vi "Doktorarbeit_Cornelius_1.10.vi"(0 "PID 1 COM":refnum<visa-resource-name>="COM3", 1 "Setpoint\n START":bool, 2 "Write to File":bool, 3 "SP 1 input (°C)":dbl=20.0 min=0.0 max=1300.0, 4 "Intervall (s)":u32=1 max=600 format="%.2f", 5 "Write/\nRead":bool=TRUE, 6 "Delay (ms)":u32=500 min=100 max=600000, 7 "Auto Tune":bool, 9 "Standby":bool, 11 "Reset\nSTOPP":bool, 12 "ON":bool caption="OFF", 13 "Get Values":bool, 15 "File Path":path) -> (8 "(°C)":dbl format="%#.3f", 14 "SP 1 is (°C)":dbl)   [LabVIEW 2010]
doc: "1. Verwendung\n\nDas Programm dient der Steuerung und Abfrage des Thermocontrollers I3252 und dem Auslesen von zwei VC 840 Messgeräten und einem Druckmessgerät Pfeiffer Single Gauge. \nDie Messgeräte werden Standardmäßig ausgelesen und erst nach Betätigung des Schalters \"Write to File\" in einer Textdatei abgespeichert. Das Eingabefeld \"Intervall\" legt den Abstand der Messpunkte fest.\nDer Setpoint für den Thermocontroller wird erst nach Betätigung des Tasters \"Setpoint START\" übernommen und angesteuert. Er wird ind den EEPROM des Gerätes geschrieben. Die Regelung kann mit Hilfe des Schalters \"Standby\" unterbrochen werden. Durch den Taster \"Reset STOPP\" kann der Setpoint aus dem EEPROM gelöscht werden.\nDie Eingabeflächen \"Constant\" und \"Thickness\" dienen der Berechnung des spezifischen Widerstands.\nDie Eingabeflächen \"User\" und \"Sample\" werden in den Header der Textdatei übernommen.\nDer Indikator \"File Path\" zeigt den aktuellen Speicherort der Textdatei an. Dieser wird nach ausschalten des Schalters \"Write to File\" gelöscht. Bei erneuten Schreiben muss ein neuer Speicherort gewählt werden. Bei Wahl desselben Speicherorts werden sämtliche bereits gespeicherte Daten gelöscht.\n\n\n2. Erläuterungen zum Blockdiagramm\n2.1 äußere Sequenz\nDie äußerte Sequenz besteht aus fünf Frames. Der erste dient der Initialisierung der Ports. Der zweite dient als Verzögerung um dem Programm genug Zeit zu geben die Ports zu öffnen. Jedoch senden die beiden VC 840 bereits Informationen an den Computer die in einem Puffer zwischengespeichert werden. Im dritten Frame wird dieser Puffer geleert. Somit kommt es zu keinem Framing Error. Desweiteren wird in diesem Frame die Startzeit der Messungen genommen. Im vierten Frame wird die eigentliche Messung und Verarbeitung der Daten durchgeführt. Die while-Schleife wird nur durch Auftreten eines Fehlers oder durch Betätigung des Stopbuttons auf dem Front Panel in der oberen linken Ecke unterbrochen. Im fünften und letzten Frame werden die Ports wieder geschlossen und beim Auftreten eines Fehlers wird das Programm automatisch gestoppt. Falls kein Fehler auftritt wird die Sequenz von vorne abgearbeitet.\n\n2.2 while-Schleife und innere Sequenz\n2.2.1 \"Event Structure\"\n2.2.1.1 Allgemein\nDer erste Frame beinhaltet ein \"Event Structure\". Dieser reagiert auf insgesamt elf verschiedene Ereignisse. Falls keines dieser Ereignisse auftreten sollte, warte die Struktur eine Millisekunde bevor die \"Event Structure\" verlassen wird. Die übrigen Ereignisse treten ein, wenn der entsprechende Kontroller eine Werteänderung erfährt.\n\n2.2.1.2 Event: Setpoint\nDieser Case besteht von außen nach innen aus einer Stacked Sequence, einer for-Loop und einer Flat Sequence die wiederum zwei \"Case Structures\" enthält. Als erstes wird bei dem Schalter \"Setpoint START\" der Blinkmodus aktiviert und bei dem Schalter \"Read Temperature\" deaktiviert. Danach folgt das eigentliche setzen des Temperatursollwerts. In der ersten Iteration wird dem Controller I3252 ein Schreibbefehl gesendet. Theoretisch kann der Setpoint in den RAM oder in den EEPROM geschrieben werden. Diese Auswahl erfolgt mit Hilfe des Schalters \"RAM\". Da das Schreiben in den RAM -Speicher aber aus diversen Gründen nicht erwünscht ist, wurde es nicht implementiert. Eine nachträgliche Implementierung ist aber leicht möglich, in dem die untere String-Konstante \"*P012\" durch \"*W012\" ersetzt wird. An diesem Befehl wird eine fünfstellige Hexadezimalzahl angehängt, die den Sollwert wiedergibt. Der Sollwert wird vorher mit zehn multipliziert, da das Komma standardmäßig nach der ersten Ziffer festgesetzt wurde (Bsp.: 800 wird gesendet um 80 einzustellen). Dieser Befehlsstrang wird an das Gerät mittels des SubVIs \"Comm_Interface\", auf welches später noch näher eingegangen wird, weitergegeben. Der durch das Gerät zurückgegebene String wird nicht verarbeitet.\nDie zweite Iteration dient dem Auslesen des eingestellten Sollwertes. Wahlweise kann der RAM- oder der EEPROM-Speicher ausgelesen werden. Die eigentliche Verarbeitung des Ausgabestrings erfolgt durch das SubVI \"Edit Setpoint\".\nDie Implementierung zur Einstellung des zweiten Setpoints erfolgt durch kopieren der ersten beiden Fälle und ersetzen der \"1\" im Befehf durch eine \"2\" (Bsp.: \"*P012\" zu \"*P022\"). Es darf aber nicht vergessen werden, dass dann ebenfalls die Anzahl der Iterationen angepasst werden muss.\nAls letztes wird der Blinkmodus des Schalters \"Setpoint START\" wieder deaktiviert.\n\n2.2.1.3 Event: Standby\nDieses Ereignis aktiviert bzw. deaktiviert als erstes den Blinckmodus des entsprechenden Schalters und sendet danach den Befehl zum aktivieren (\"*D03\") oder zum deaktivieren (\"*E03\") des Standbymodus an den Thermocontroller.\n\n2.2.1.4 Event: Set Command \nDer in das Feld \"Command shall be\" eingegebene Befehl wird an den Thermocontroller übermittlet. Die korrekte Form des Befehls ist im \"Communication Manuel\" nachzuschlagen. Das \"*\"-Zeichen wurde allerdings schon implementiert und muss somit nicht mit eingegeben werden.\n\n2.2.1.5 Event: Reset\nIn der ersten Iteration wird der Reset-Befehl an den Thermocontroller gesendet. In Folge wird der gesamte EEPROM-Speicher gelöscht. Deshalb wird in der zweiten Iteration der Setpoint aktualisiert. Dieser Befehl hat keinen Einfluss auf den RAM-Speicher. Die anschließende Wartezeit ist auf vier Sekunden festgesetzt und wurde empirisch ermittelt. Diese Zeit benötigt das Gerät um den Reset durchzuführen und für die Kommunikation wieder zur Verfügung zu stehen.\n\n2.2.1.6 Event: Auto Tune\nEs ist festgeschrieben, dass der Setpoint für die \"Auto Tune\"-Funktion wenigstens 20°C über der aktuellen Temperatur liegt. Deshalb wird zunächst der aktuelle Temperaturwert ausgelesen. Im zweiten Schritt werden zu diesem Wert zwanzig addiert und der Setpoint wird in den RAM-Speicher geschrieben. Das Schreiben in diesen Speicher ist nötig, da die \"Auto Tune\"-Funktion\" erst nach einem Reset startet. Im dritten Schritt wird der eigentliche Befehl für den \"Auto Tune\" gesendet (siehe dazu \"Communication Manuel\" S.27). Als vierte und letzte Iteration der for-Schleife folgt der bereits erwähnte Reset-Befehl. Der Temperatursollwert, der im RAM-Speicher eingetragen ist, muss zum Schluss wieder auf 0°C gesetzt werden. Die Zeit für die Ausführung des \"Auto Tune\"-Befehls wurde empirisch ermittelt und 45 s festgesetzt.\n\n2.2.1.7 Event: Write LOW/HI\nDieses Ereignis setzt die am Analogausgang anliegende Spannung fest. Normalerweise beträgt dieser Spannungswert 0-10 V. Das angeschlossene Netzteil verträgt aber maximal nur 2,3 V. Aus diesem Grund wird der \"%HIGH\" auf 23 gesetzt. Somit beträgt die maximal anliegende Spannung nur noch 23% von der maximal möglichen, d.h 2,3V. Ein niedrigerer Wert ist jederzeit möglich, genauso wie ein höherer für den Parameter \"%LOW\". Diese werden zunächst nacheinander in den RAM-Speicher geschrieben und anschließend wieder ausgelesen.\n\n2.2.1.8 Event: Set PID\nDie Werte für den PID-Regler können sowohl mit Hilfe der \"Auto Tune\"-Funktion, als auch manuell eingestellt werden. Es wird wiederum zwischen dem Schreiben in den RAM- und dem EEPROM-Speicher unterschieden. Zunächst werden die Werte für \"P\", \"I\" und \"D\", in dieser Reihenfolge, gesetzt und danach die aktuellen Werte ausgelesen.\n\n2.2.1.9 Event: Get Values\nDieses Ereignis hat zur Folge, dass die Werte für \"P\", \"I\", \"D\", \"%LOW\", \"%HIGH\" und des Setpoints wahlweise aus dem RAM- oder EEPROM-Speicher gelesen werden. Die aktuellen Werte werden nicht nur in die entsprechenden Anzeigefelder übernommen, sondern auch in die entsprechenden Eingabefelder, mit Ausnahme des Temperatursollwerts. \n\n2.2.1.10 Event: RAM\nPrinzipiell kann zwischen dem Schreiben in den RAM- oder EEPROM-Speicher des Thermocontrollers gewählt werden. Die entsprechende Schalterposition auf dem Frontpanel zeigt den aktuell verwendeten Speicher an. Die Anzeigewerte werden bei jedem Umschalten aktualisiert und sind im entsprechenden Speicher eingetragen. Die Implementierung ist identisch mit der des Ereignisses \"Get Values\". Es gilt zu beachten, dass die Werte für \"%LOW\" und \"%HIGH\" nur in den RAM-Speicher geschrieben werden können und somit auch nur aus diesem ausgelesen werden können.\n\n2.2.1.11 Event: Set Gauge to Zero\nMit Hilfe der SubVIs \"Get Pressure\" und \"Offset Display\" werden die Werte für den alten und den neuen Offset und der durch den zweiten Drucksensor ermittelt Druck ermittelt. \n\n2.2.1.12 Event: Write to File\nSollte der Schalter \"Write to File\" aktiviert werden, d.h. Schalterposition oben, so wird zunächst durch das SubVI \"Header\" ein Header für die unter \"File Path\" definierte Datei angelegt. Alle Werte, die bereits in der entsprechenden Datei stehen, werden dabei gelöscht.\n\n2.2.2 \"Timed Structures\"\nIm dritten Frame der inneren Sequenz werden die Werte für Zeitpunkt, Temperatur, Spannung, Strom und Druck ermittelt. Damit die Werte zum gleichen Zeitpunkt aufgenommen werden, werden \"Timed Sequences\" eingesetzt. Mit dem entsprechenden Schalter auf dem Front Panel unter dem Tab \"Settings\" kann gewählt werden, ob das entsprechende Gerät ausgelesen werden soll oder nicht. Die einzelnen Sequenzen werden parallel abgearbeitet, womit die Prozesszeit von diesem Frame durch der zeitintensivsten Sequenz abhängt. Dies ist in aller Regel das Auslesen der Temperatur, da ein \"Delay\" von 500 ms oder größer benötigt wird, um den Controller ordentlich ansprechen zu können.\nDie Systemzeit wird durch das SubVI \"System Time in Seconds\" in Sekunden umgerechnet und der in dem Parameter \"Starttime\" gespeicherte Wert wird abgezogen. Somit werden die Sekunden seit dem Start des Programms gezählt.\n\n2.2.3 restlichen Frames\nIm zweiten Frame wird das Intervall zwischen den einzelnen Messwerten festgelegt. Dabei wird der Wert des Parameters \"Delay\" abgezogen. Dieser Wert beträgt im Normalfall 500 ms und ist somit nicht vernachlääsigbar.\nDer Vierte Frame beinhaltet die Umrechnung des Temperatur-Strings in einen Temperaturwert durch das SubVI \"Edit Tmperature\", die Berechnung des spezifischen Widerstands durch das SubVI \"Resistivity Calculation\" und die Überprüfung des Druckwerts. Auch werden die neu gewonnen Werte in das entsprechende Shift-Register übernommen. Falls der Druckwert einen in dem Parameter \"Pressure Limit (mbar)\" festgelegten Grenzwert überschreiten sollte, wird der Thermocontroller automatisch in den Standby-Modus versetzt. Des Weiteren wird der Schalter \"Standby\" solange gesperrt, wie der Druck oberhalb des Grenzwertes liegt. Wenn der Druck wieder unter den Grenzwert gesunken ist, wird der Standby-Befehl nicht automatisch aufgehoben, sondern muss vom Benutzer durch Betätigung des entsprechenden Schalters gegeben werden.\nIm fünften Frame werden die Diagramme erstellt. Dabei wird jedes Mal von neuem das gesamte Shift-Register als Graph dargestellt. Weiterhin werden die Messwerte in ein 1D-Array geschrieben.\nDer sechste und letzte Frame beinhaltet den eigentlich Schreibvorgang der Messwerte in eine Textdatei und die Überprüfung ob ein Fehler vorliegt.\n\n2.3 SubVIs\n2.3.1 Allgemein\nDie SubVIs für die Messgeräte VC840 und das Druckmessgerät wurden aus anderen Quellen übernommen. \n\n2.3.2 \"Header\"\nIn den Header wird zunächst das aktuelle Datum und die aktuelle Zeit übernommen. Die ausgewählte Datei wird dabei überschrieben. Danach wird der Name des Benutzers und der Probe übernommen. Zum Schluss werden die Einheiten in einer Reihe, durch einen Tabulator getrennt, in den Header geschrieben.\n\n2.3.3 \"I3252 Comm Interface\"\nDieses VI stellt die Kommunikation mit dem Thermocontroller her und gibt den Ausgabe-String zurück.\n\n2.3.4 \"I3252 Edit Setpoint\"\nIm Ausgabe-String vom Thermocontroller ist an der vierten Stelle die Stelle des Dezimalpunktes verschlüsselt. Dieses Hexadezimalzahl wird herausgefiltert und an ein \"ENUM Controller\" übergeben. Dieser weist der Hexadezimalzahl eine Nummer zu, mit welcher ein Wert aus einem Array entnommen wird. Dieser Wert dient als Quotient. Der tatsächliche Wert kann somit errechnet werden.\n\n2.3.5 \"I3252 Edit Temperature\"\nDer Temperatur-String, der vom Thermocontroller zurückgegeben wird, wird in eine Dezimalzahl umgewandelt. Manchmal kommt es aus zu Dropouts, die durch dieses Programm herausgefiltert werden. Der letzte Wert wird dabei in einer \"Feedback Node\" gehalten unter der Annahme, dass sich der Temperaturwert nicht sprunghaft ändert.\n\n2.3.6 \"Resistivity Calculation\"\nDer spezifische Widerstand wird nach folgender Formel ausgerechnet. Dabei entspricht t der Dicke der Probe und C ist eine Konstante.\nrho=C*pi*t*U/(ln( 2)*I)\n\n2.3.7 \"System Time in Seconds\"\nZunächst wird die aktuelle Systemzeit ausgelesen. Danach wird diese in Stunden, Minuten und Sekunden aufgeteilt, alles in Sekunden umgerechnet und letztendlich addiert."
uses:
  <vilib>/Platform/TimedLoop/XDataNode/XDataNode.xnode
  <vilib>/Platform/TimedLoop/XDataNode/timing_clust.ctl
  <vilib>/Platform/TimedLoop/XDataNode/nitl_modes.ctl
  <vilib>/Platform/TimedLoop/XDataNode/wakeup.ctl
  <vilib>/Instr/_visa.llb/VISA Configure Serial Port (Instr).vi
  <vilib>/Platform/TimedLoop/scheduler/LVUserAPI/_suppVIs/Create_1kHz_TSource.vi
  <vilib>/Utility/file.llb/Write To Spreadsheet File (DBL).vi
  <vilib>/Platform/TimedLoop/XDataNode/XDNodeRunTimeDep.lvlib
  Labview 8 Tutorial/Dual Gauge/Dual Gauge.lvlib
panel:
  out "appended array":dbl[](array[numeric])
  in  "Tab Control":T1(tab)
  in  "Thickness (nm)":dbl min=0.0
  in  "4PP constant":dbl min=0.0 max=5.0
  in  "Sample":string
  in  "User":string
  out "Sample holder (Type-K Thermocouple)":cluster{dbl[], dbl[]}(graph)
  out "current time (s)":dbl
  out "data logger intervall (s)":dbl
  out "loop time (s)":ext
  in  "stop":bool
  out "Main Chamber (PG-1)":cluster{dbl[], dbl[]}(graph)
  out "Pressure Gauge 1#1":dbl format="%#_4e"
  out "Loadlock (PG-3)":cluster{dbl[], dbl[]}(graph)
  out "Pressure Gauge 1#2":dbl format="%#_3e"
  out "Pressure Gauge 2#1":dbl format="%#_3e"
  out "Pressure OpenPort":cluster{dbl[], dbl[]}(graph)
  out "Pressure Gauge 2#2":dbl caption="current"
  out "Pirani (VVP1 Scroll)":cluster{dbl[], dbl[]}(graph)
  out "status 2":bool caption="Status"
  out "code 2":i32 caption="Code"
  out "code":i32 caption="Code"
  out "status":bool caption="Status"
  in  "Set Gauge to Zero":bool
  out "Status Gauge 1#2":i32(ring) items=["data OK", "underrange", "overrange", "sensor error", "sensor off", "no sensor", "ID error"]
  out "Pressure Gauge 1#2":dbl format="%.3e"
  out "Pressure Gauge 1#1":dbl format="%.3e"
  out "Status Gauge 1#1":i32(ring) items=["data OK", "underrange", "overrange", "sensor error", "sensor off", "no sensor", "ID error"]
  in  "TPG 1 COM":refnum<visa-resource-name>="COM1"
  in  "Pressure Limit (mbar)":dbl=1.0 min=0.0 max=1100.0
  out "Current Offset (mbar)":dbl
  in  "ON (TPG 2)":bool caption="OFF"
  in  "ON (TPG 1)":bool=TRUE caption="OFF"
  in  "ON":bool caption="OFF"
  in  "VC 840 2":refnum<visa-resource-name>="COM4"
  out "Reading 2":dbl format="%_4f"
  out "Mode 2":enum16{"?", "Diode", "Beep", "DC", "AC"}(ring)
  out "Unit 2":string
  in  "VC 840 1":refnum<visa-resource-name>="COM4"
  out "Reading 1":dbl format="%_4f"
  out "Mode 1":enum16{"?", "Diode", "Beep", "DC", "AC"}(ring)
  out "Unit 1":string
  out "Status 1":T2
  out "Status 2":T2
  in  "ON":bool caption="OFF"
  out "% HIGH Istwert":u32
  out "% LOW Istwert":u32
  in  "% High Sollwert":u32=23 max=24
  in  "% LOW Sollwert":u32 max=25
  in  "RAM":bool=TRUE caption="EEPROM"
  out "D (Rate) IstWert":u32
  out "I ( Reset1) Istwert":u32
  out "P (PB1) Istwert":u32 caption="actual value"
  in  "D (Rate) Sollwert":u32 max=3999
  in  "I ( Reset1) Sollwert":u32 max=3999
  in  "P (PB1) Sollwert":u32 caption="set value" max=9999
  in  "Set Command":bool
  in  "Set PID":bool
  in  "Write LOW/HI":bool
  in  "Flow Control":u16(ring) items=["None"=0, "XON/XOFF"=1, "RTS/CTS"=2, "DTR/DSR"=4]
  in  "Stop Bits":u16(ring)=10 items=["1.0"=10, "1.5"=15, "2.0"=20]
  in  "Parity":u16(ring)=1 items=["None", "Odd", "Even", "Mark", "Space"]
  in  "Data Bits":u16=7 min=5 max=8 step=1
  in  "Baud Rate":u32=9600
  out "Command output":string
  in  "Command input":string
  in  "TPG 2 COM":refnum<visa-resource-name>="COM4"
  out "Pressure Gauge 2#2":dbl format="%.3e"
  out "Pressure Gauge 2#1":dbl format="%.3e"
  out "Status Gauge 2#2":i32(ring) items=["data OK", "underrange", "overrange", "sensor error", "sensor off", "no sensor", "ID error"]
  out "Status Gauge 2#1":i32(ring) items=["data OK", "underrange", "overrange", "sensor error", "sensor off", "no sensor", "ID error"]
  out "Current":cluster{dbl[], dbl[]}(graph)
  out "Voltage":cluster{dbl[], dbl[]}(graph)
  out "Voltage (V)":dbl format="%.4e"
  out "Current (A)":dbl format="%.4e"
  out "Resistivity":cluster{dbl[], dbl[]}(graph)
  out "Resistivity (Ohm*cm)":dbl format="%.3e"
  # "set \nvalue"
  # "actual \nvalue"
  # "T (°C)"
  # "mbar"
  # "mbar"
  # "mbar"
  # "mbar"
  # "Pressure Measurement \n(Pfeiffer TPG261)"
  # "PID Controller (Omega Newport i3252)"
  # "limit (mbar)"
  # "Multimeter\n#1 (VC 840)"
  # "Multimeter\n#2 (VC 840)"
  # "P"
  # "I"
  # "D"
  # "% Low"
  # "% High"
  # "Authors:  Daniel Schuster (sir-dan@web.de)\n                 Steffen Cornelius (s.cornelius@hzdr.de)\n                 Nico Spahn (x)\n\n                 premade SubVIs for readout of Pfeiffer gauge and VC840 Multimeters were used\n                 SubVI \"I3252_Comm_Interface\" is based on a modified Labview example\n\nRelease:  v1.0    \n\nVersion History:\n\nv1.1  -    28.06.2011\n             - Format des Files geändert von %.3f auf %g\n             - maximale Eingabewerte für PID begrenzt\nv1.2  -    12.07.2011\n             - Anzeige p,rho, U, V auf Scientific geändert\n             - y-Achse p,rho auf Log geändert\n             - numerische Zeitanzeige hinzugefügt\n             - 4PP Constant: pi/ln(2)=4,532 set as the default value\nv1.3  -    25.07.2011\n             - Zeitvariable auf EXT geändert, um Sprünge in Diagrammen loszuwerden\nv1.4  -   27.07.2011\n             - ALLE Variablen auf DBL zurückgesetzt wegen Formatierungsproblem im File\n             - Zeitberechnung neu gemacht (Tick count differenzen) -> Zeitsprünge korrigiert ?\n             - Delay/Intervall überarbeitet\nv1.5  -   05.12.2012\n                - Austausch der alten Pfeifer SubvIs durch neue -> nun alle 4 Kanäle des DualGauge\n                                                                                                         Controllers gleichzeitig auslesbar\n                - neue Pfeiffer SubVIs verwendet in Druckwertauslesung und Offset Berechnung des Baratron\n                  Druckes (COM5 Sensor1)\n                - Neuarragement des GUI -> FullRange und Baratron neben Temperatur auf Haupseite zu sehen\n                                                                   Pirani und OpenPort auf Meas.2 zu sehen\n                                                                   Diagnose Seite umfasst nun auch Widerstandsdiagramm\n                - Änderungen der Settingseite -> nun alle 4 Drucksensoren mit aktuellem Messwert und Gerätestatus\n                                                                           zu sehen\n                - The readout of the PID-Temperature Controller and the VC840 Multimeters was not modified\nv1.73  -  18.10.2013\n                - Layout Änderungen\nv.1.8   -  19.01.2014\n                - Änderung Layout Settings Tab\n                - Trennung der beiden TPG Dual Gauge Controls\n                -"
  # "Version 1.73    - last change 18.10.2013"
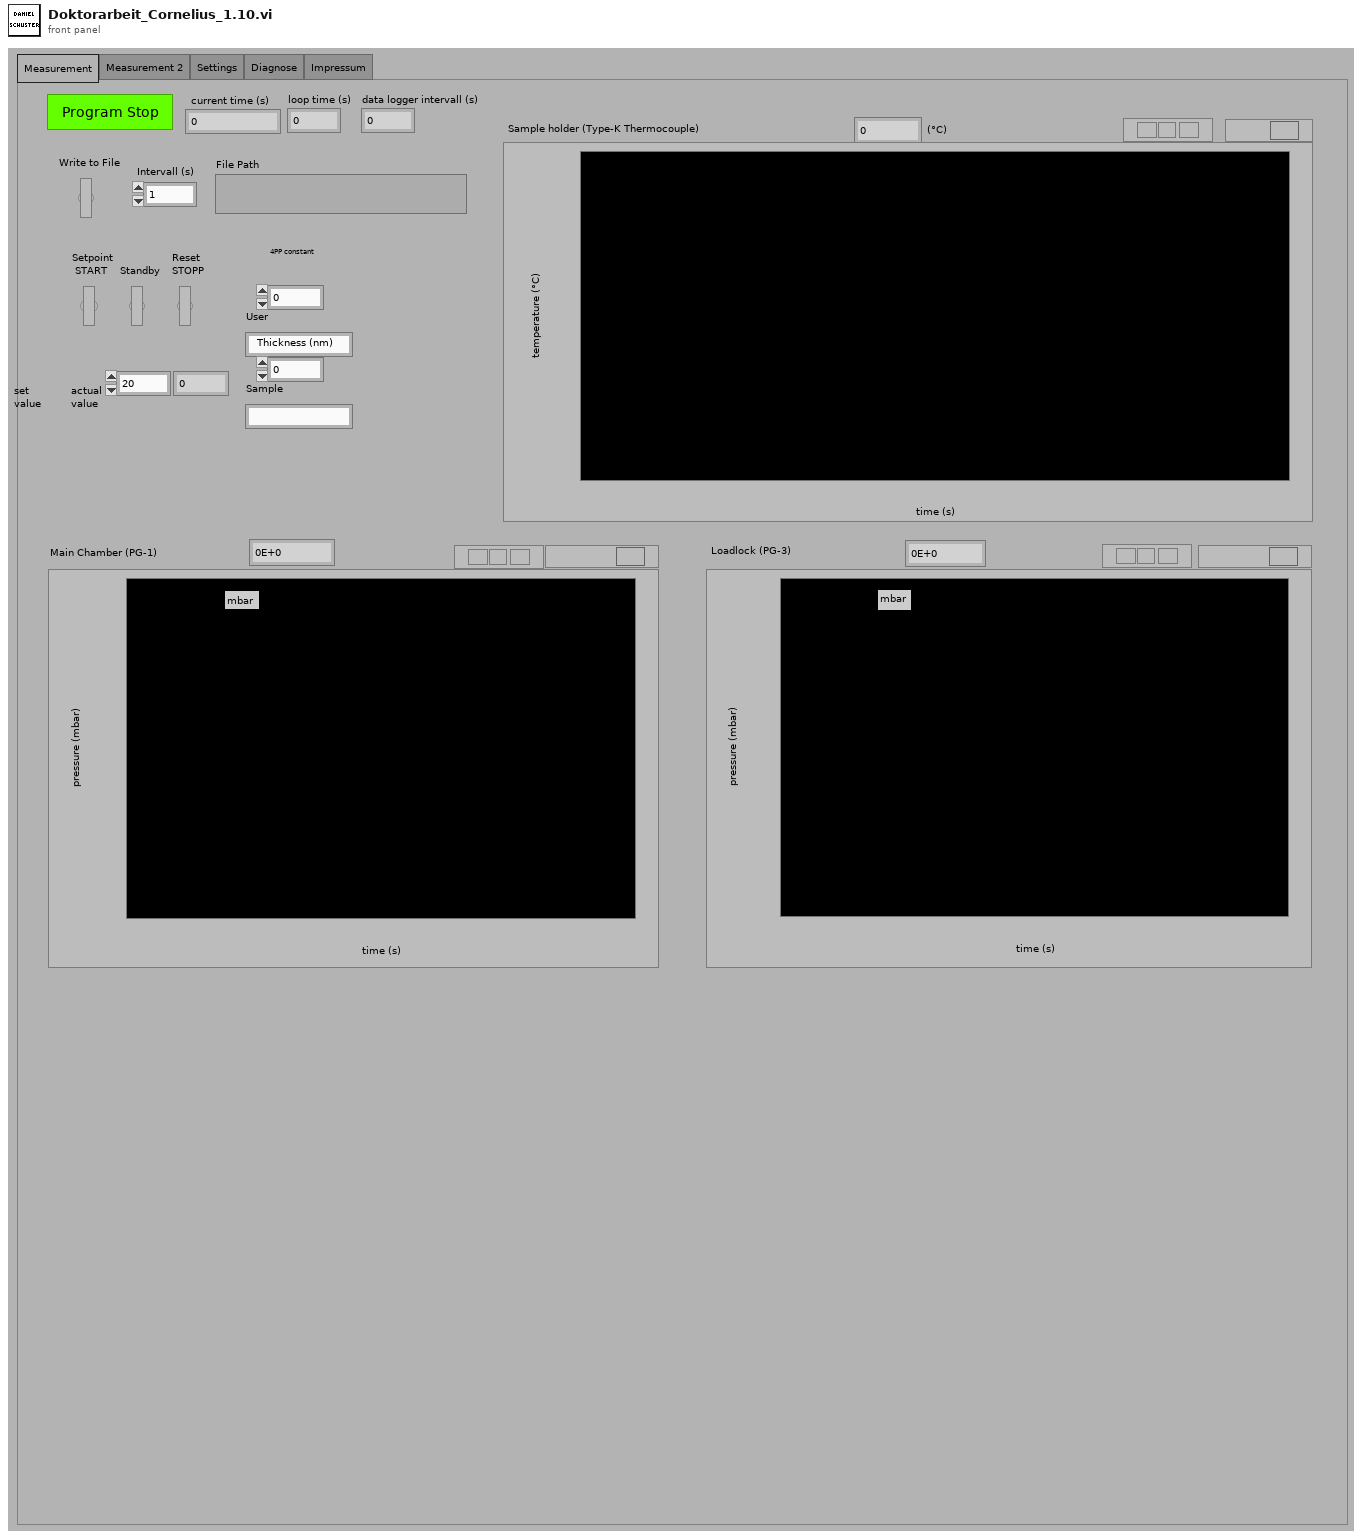
[diagram p1: front panel]
types:
  T1 = enum32{"Measurement", "Measurement 2", "Settings", "Diagnose", "Impressum"}
  T2 = cluster{"Low Bat":bool, "Auto":bool, "Delta":bool, "Hold":bool, "RS232":bool}
  T3 = typedef "XDNodeRunTimeDep.lvlib/timing_clust.ctl" = cluster{"Expected End [f-1]":u64, "Actual End [f-1]":u64, "Finished Late? [f-1]":bool, "Expected End [i-1]":u64, "Actual End [i-1]":u64, "Finished Late? [i-1]":bool, "Expected Start [i]":u64, "Actual Start [i]":u64, "Expected Start [f]":u64, "Actual Start [f]":u64, "Source Name":string, "Structure Name":string, "Period":i64, "Deadline":i64, "Offset":i64, "Start":i64, "Priority":i32, "Timeout":i32, "Mode":T4, "Wakeup Reason":T5, "Error":errorcluster, "Source Type":string, "Secondary Source Type":string, "Global End Time":u64, "Global Start Time":u64, "Frame Duration":u64, "Iteration Duration":u64, "Assigned CPU":i32, "I/O Scan Engine Mode":u32}
  T4 = typedef "XDNodeRunTimeDep.lvlib/nitl_modes.ctl" = enum32{"No Change", "Process missed periods, maintain original phase", "Discard missed periods, maintain original phase", "Process missed periods, ignore original phase", "Discard missed periods, ignore original phase"}
  T5 = typedef "XDNodeRunTimeDep.lvlib/wakeup.ctl" = enum32{"Normal", "Aborted", "Asynchronous wakeup", "Timing source error", "Timed loop error", "Timeout"}
  T6 = enum8{"Enabled", "Disabled", "Disabled and Grayed Out"}
  T7 = cluster{"VISA resource name out":refnum<visa-resource-name>, "error out":errorcluster, "Delay (ms)":u32, "Write/\nRead":bool}
  T8 = cluster{"TPG 2 COM":refnum<visa-resource-name>, "error out":errorcluster}
  T9 = cluster{"COM out":refnum<visa-resource-name>, "Cluster (Ausgang)":errorcluster}
  T10 = cluster{"Pressure Gauge#1":dbl, "Pressure Gauge#2":dbl}
  T11 = cluster{"TPG 1 COM":refnum<visa-resource-name>, "error out":errorcluster}
  T12 = cluster{"COM out":refnum<visa-resource-name>, "error out":errorcluster, "COM out":refnum<visa-resource-name>, "error out":errorcluster}
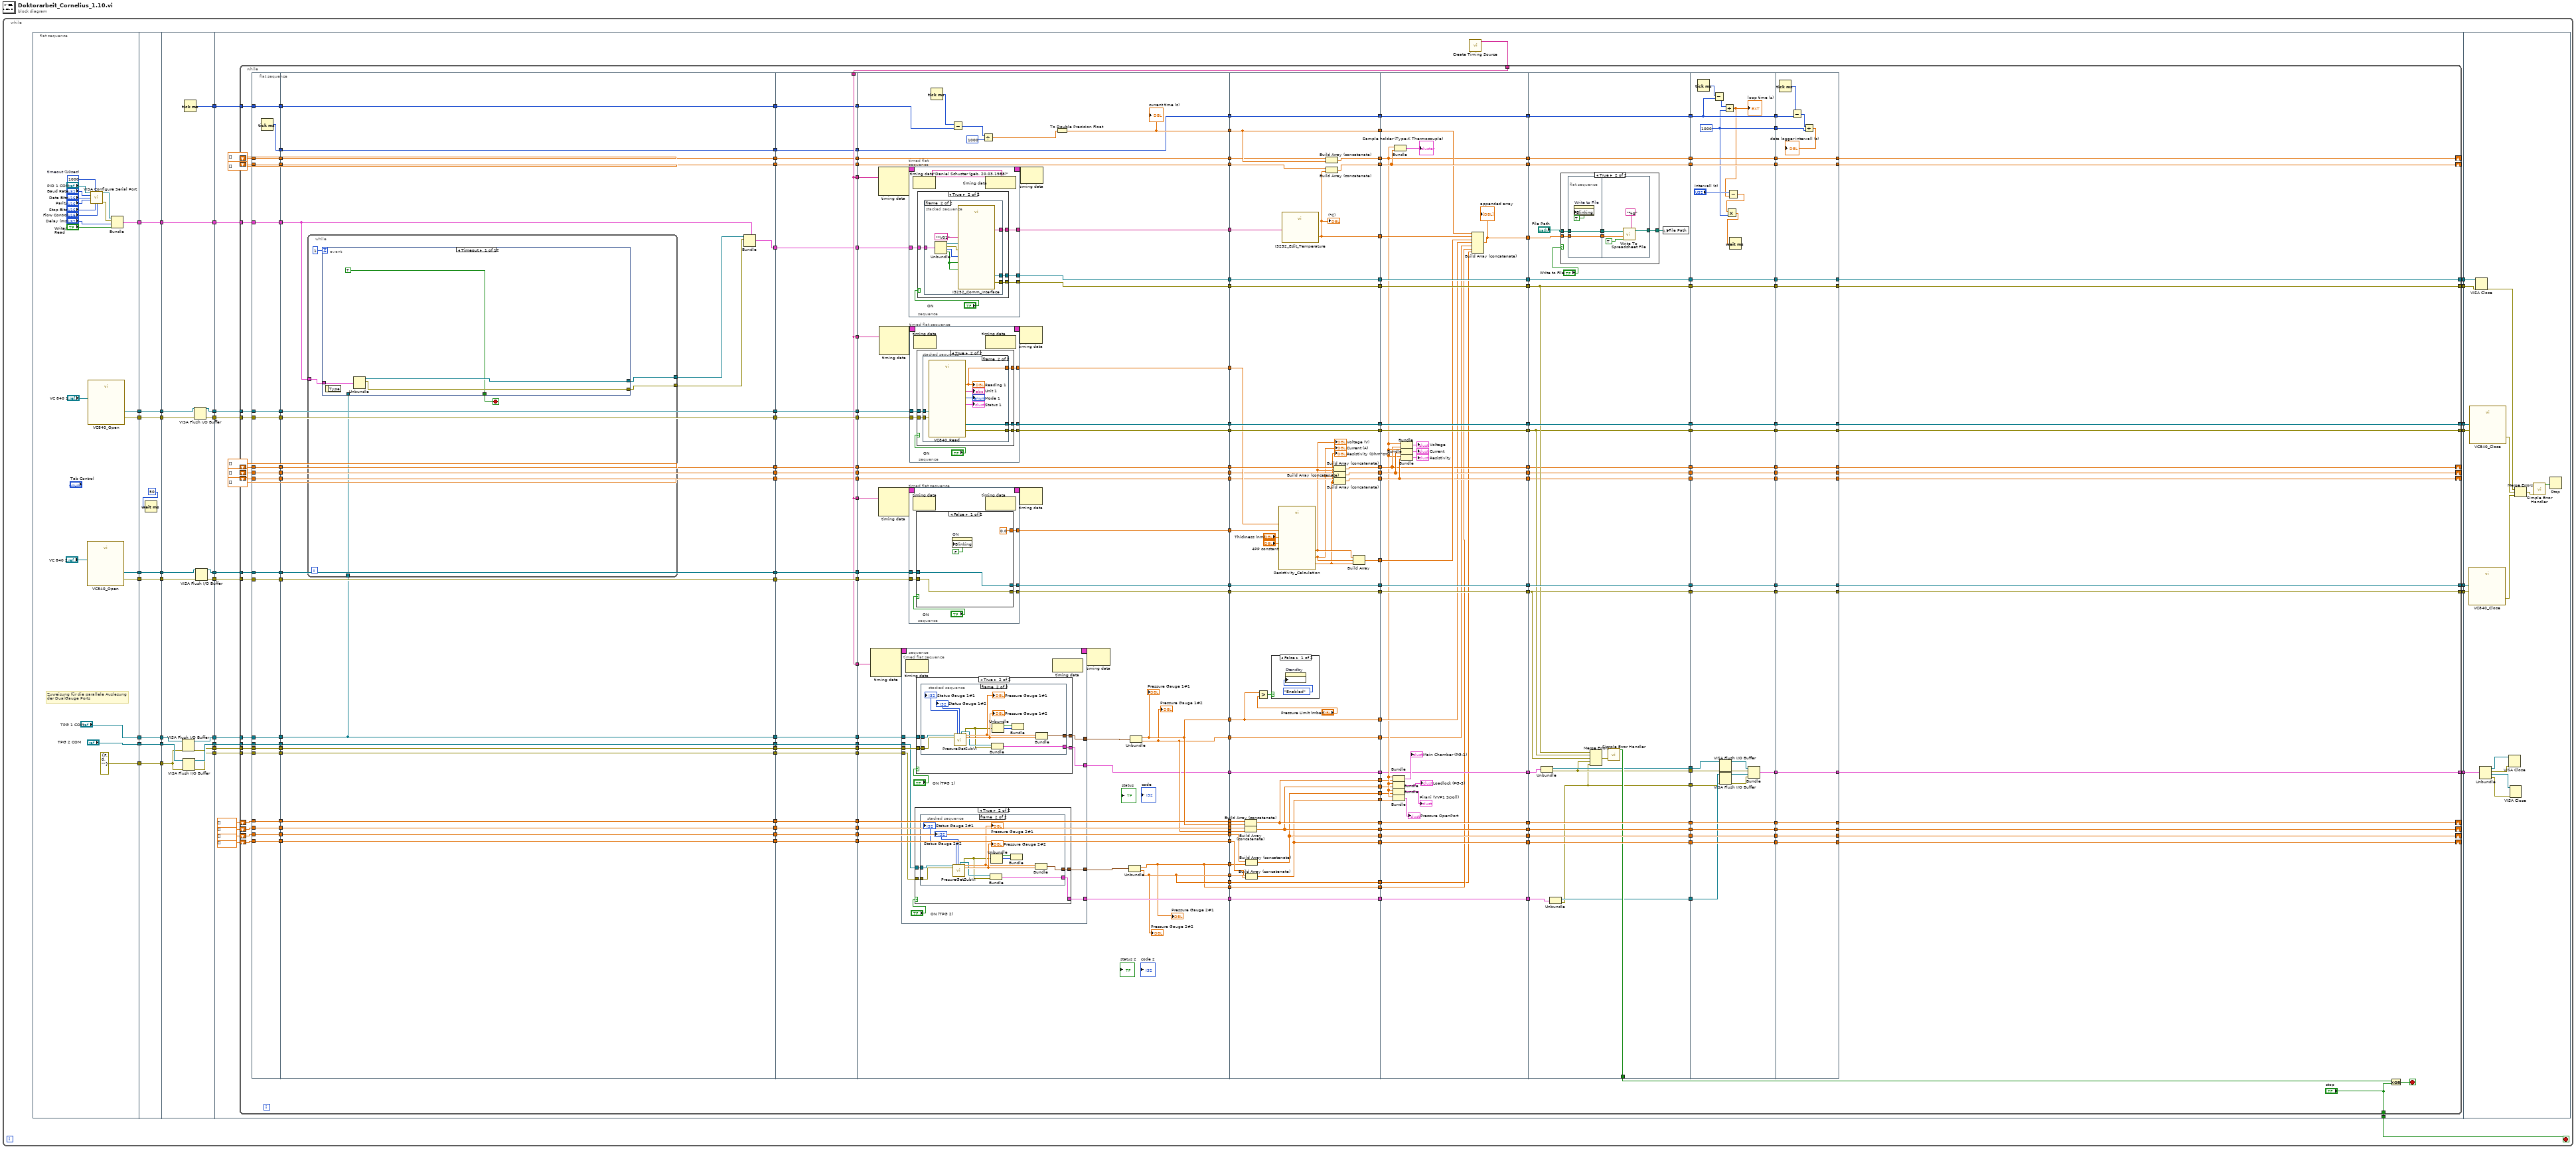
[diagram p0: block diagram]
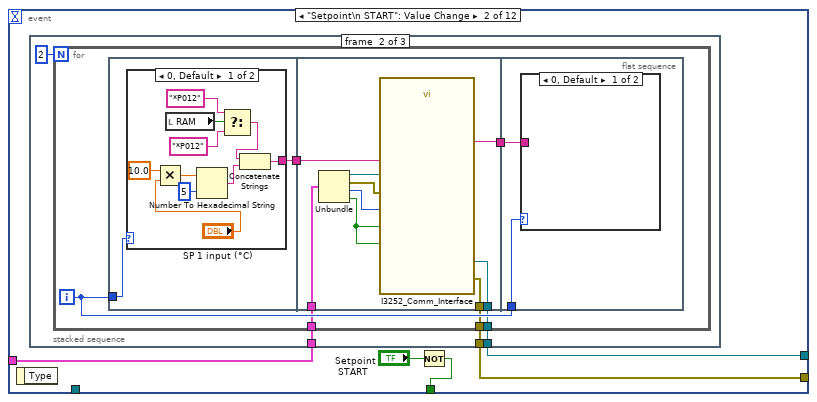
[diagram p2: hidden frame]
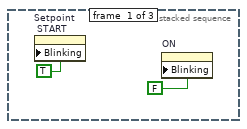
[diagram p3: hidden frame]
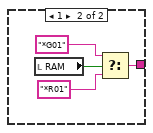
[diagram p4: hidden frame]
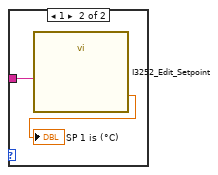
[diagram p5: hidden frame]
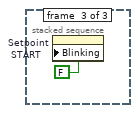
[diagram p6: hidden frame]
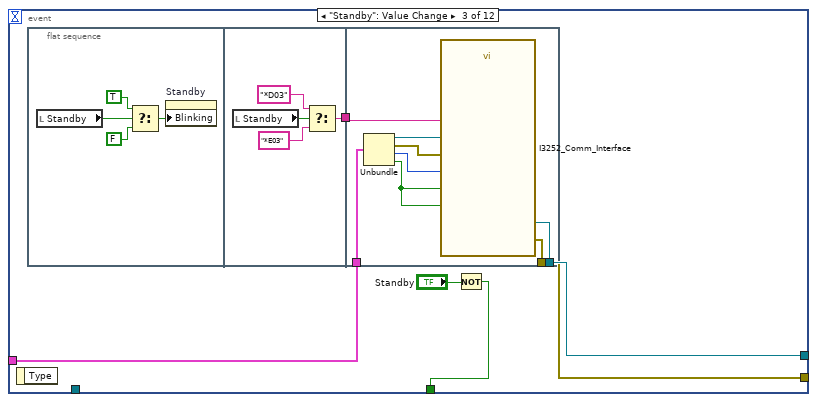
[diagram p7: hidden frame]
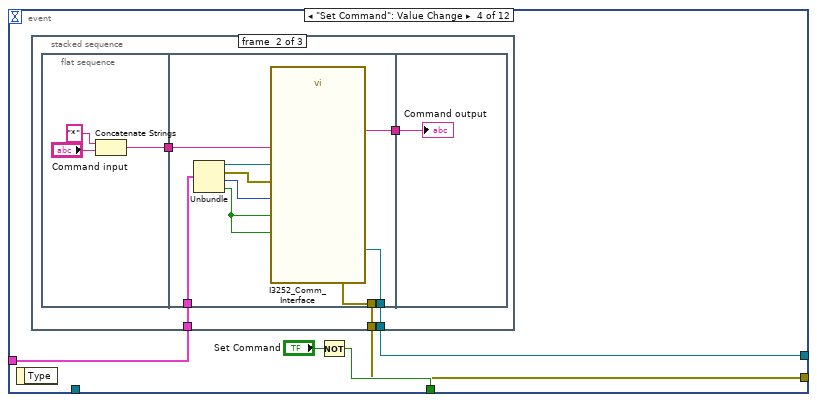
[diagram p8: hidden frame]
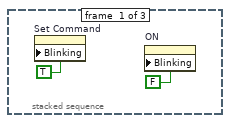
[diagram p9: hidden frame]
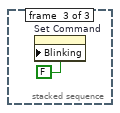
[diagram p10: hidden frame]
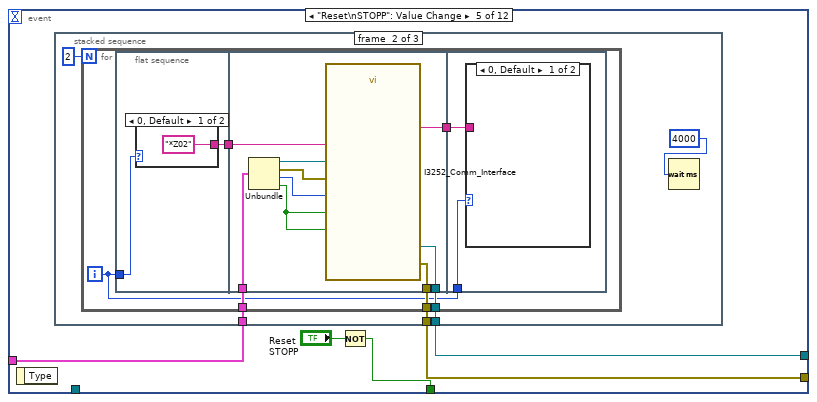
[diagram p11: hidden frame]
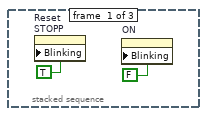
[diagram p12: hidden frame]
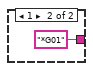
[diagram p13: hidden frame]
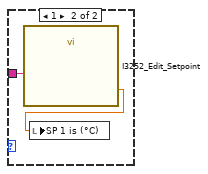
[diagram p14: hidden frame]
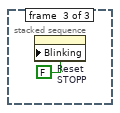
[diagram p15: hidden frame]
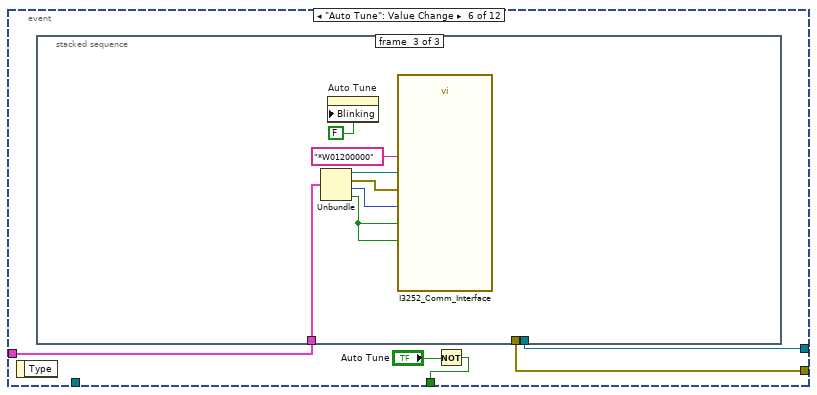
[diagram p16: hidden frame]
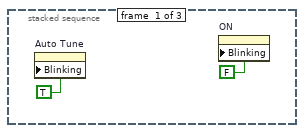
[diagram p17: hidden frame]
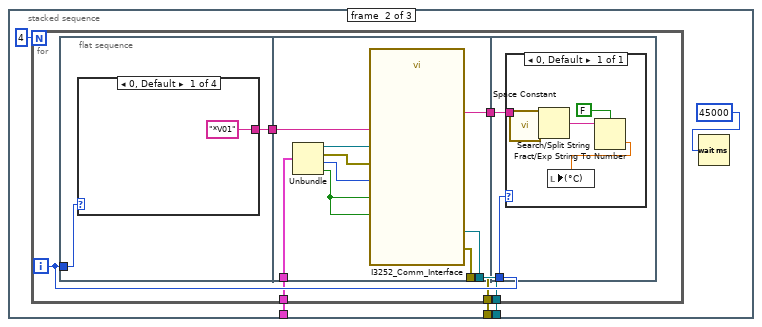
[diagram p18: hidden frame]
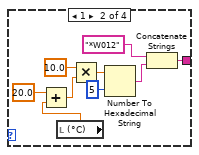
[diagram p19: hidden frame]
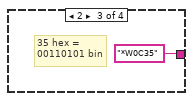
[diagram p20: hidden frame]
diagram:
  n1 = while {
    stop <- w6 stop-if-true
    n2 = flat-sequence {
      tunnel: [w54] -> w34
      tunnel: [w55] -> w33
      tunnel: [w40] -> w32
      tunnel: [w53] -> w31
      tunnel: [w52] -> w30
      tunnel: ["TPG 1 COM"] -> w29
      tunnel: ["TPG 2 COM"] -> w28
      tunnel: [errorcluster {"status"=FALSE, "code"=0, "source"=""} ("Fehler (Eingang)")] -> w3
      tunnel: w34 -> [w64]
      tunnel: [w64] -> w27
      tunnel: w33 -> [w63]
      tunnel: [w63] -> w26
      tunnel: w32 -> [w62]
      tunnel: [w62] -> w25
      tunnel: w31 -> [w61]
      tunnel: [w61] -> w24
      tunnel: w30 -> [w60]
      tunnel: [w60] -> w23
      tunnel: [w58] -> w22
      tunnel: w29 -> [w58]
      tunnel: [w57] -> w21
      tunnel: w28 -> [w57]
      tunnel: [w56] -> w4
      tunnel: w3 -> [w56]
      tunnel: w27 -> [w75]
      tunnel: [w74] -> w20
      tunnel: w26 -> [w76]
      tunnel: [w73] -> w19
      tunnel: w25 -> [w81]
      tunnel: [w81] -> w18
      tunnel: w24 -> [w78]
      tunnel: [w79] -> w17
      tunnel: w23 -> [w77]
      tunnel: [w80] -> w16
      tunnel: [w72] -> w15
      tunnel: [w70] -> w14
      tunnel: w22 -> [w71]
      tunnel: [w69] -> w13
      tunnel: w21 -> [w68]
      tunnel: w4 -> [w67]
      tunnel: [w66] -> w2
      tunnel: [w65] -> w1
      tunnel: w20 -> [w109]
      tunnel: w19 -> [w108]
      tunnel: w18 -> [w107]
      tunnel: w17 -> [w105]
      tunnel: w16 -> [w104]
      tunnel: [w103] -> w12
      tunnel: [w102] -> w11
      tunnel: [w101] -> w10
      tunnel: [w100] -> w9
      tunnel: [w99] -> w8
      tunnel: [w98] -> w7
      tunnel: w15 -> [w92]
      tunnel: w14 -> [w91]
      tunnel: w13 -> [w90]
      tunnel: [w85] -> w6
      tunnel: [w84] -> w5
      tunnel: w2 -> [w83]
      tunnel: w1 -> [w82]
      tunnel: w12 -> [w1315]
      tunnel: w11 -> [w1314]
      tunnel: w10 -> [w1317]
      tunnel: w9 -> [w1316]
      tunnel: w8 -> [w1319]
      tunnel: w7 -> [w1318]
      tunnel: w5 -> [w1312]
      frame #0 {
        w41 = u32 1000  # timeout (10sec)
        # "Zuweisung für die parallele Auslesung\nder DualGauge Ports"
        n3 = call "VC840_Open.vi"("VISA resource name"="VC 840 2") -> ("error out"=w52:errorcluster, "VISA resource name out"=w53:refnum<visa-resource-name>)  [unwired: 1 in, 8 out]
        n4 = call "VC840_Open.vi"("VISA resource name"="VC 840 1") -> ("error out"=w55:errorcluster, "VISA resource name out"=w54:refnum<visa-resource-name>)  [unwired: 1 in, 8 out]
        n5 = call-poly "VISA Configure Serial Port"("VISA resource name"="PID 1 COM", "timeout (10sec)"=w41, "baud rate (9600)"="Baud Rate", "data bits (8)"="Data Bits", "parity (0:none)"="Parity", "stop bits (10: 1 bit)"="Stop Bits", "flow control (0:none)"="Flow Control") -> ("VISA resource name out"=w50:refnum<visa-resource-name>, "error out"=w51:errorcluster)  [unwired: 2 in, 5 out]
        n6 = Bundle("VISA resource name out"=w50, "error out"=w51, "Delay (ms)"="Delay (ms)", "Write/\nRead"="Write/\nRead") -> (w40:T7)  [unwired: 1 in]
      }
      frame #1 {
        n7 = Wait (ms)(milliseconds to wait=u32 50) -> ()  [unwired: 1 out]
      }
      frame #2 {
        n8 = VISA Flush I/O Buffer(VISA resource name=w71, error in (no error)=w67) -> (VISA resource name out=w70:refnum<visa-resource-name>, error out=w66:errorcluster)  [unwired: 1 in]
        n9 = VISA Flush I/O Buffer(VISA resource name=w68, error in (no error)=w67) -> (VISA resource name out=w69:refnum<visa-resource-name>, error out=w65:errorcluster)  [unwired: 1 in]
        n10 = Tick Count (ms)() -> (millisecond timer value=w72:u32)
        n11 = VISA Flush I/O Buffer(VISA resource name=w75, error in (no error)=w76) -> (VISA resource name out=w74:refnum<visa-resource-name>, error out=w73:errorcluster)  [unwired: 1 in]
        n12 = VISA Flush I/O Buffer(VISA resource name=w78, error in (no error)=w77) -> (VISA resource name out=w79:refnum<visa-resource-name>, error out=w80:errorcluster)  [unwired: 1 in]
      }
      frame #3 {
        n13 = call-poly <vilib>:"Create Timing Source.vi"() -> ("name (out)"=w106:string)  [unwired: 10 in, 1 out]
        n14 = while {
          tunnel: w109 -> [w328]
          tunnel: w108 -> [w327]
          tunnel: w107 -> [w326]
          tunnel: w106 -> [w319]
          tunnel: w105 -> [w312]
          tunnel: w104 -> [w311]
          tunnel: [w307] -> w103
          tunnel: [w306] -> w102
          tunnel: [w304] -> w101
          tunnel: [w302] -> w100
          tunnel: [w300] -> w99
          tunnel: [w298] -> w98
          shift-right: [w271] -> _
          shift-left: dbl[] [] -> [w276]
          shift-right: [w249] -> _
          shift-left: dbl[] [] -> [w284]
          shift-right: [w273] -> _
          shift-left: dbl[] [] -> [w280]
          shift-right: [w246] -> _
          shift-left: dbl[] [] -> [w283]
          shift-right: [w243] -> _
          shift-left: dbl[] [] -> [w282]
          tunnel: w92 -> [w237]
          tunnel: w91 -> [w193]
          tunnel: w90 -> [w189]
          shift-right: [w147] -> _
          shift-left: dbl[] [] -> [w177]
          shift-right: [w145] -> _
          shift-left: dbl[] [] -> [w175]
          shift-right: [w143] -> _
          shift-left: dbl[] [] -> [w173]
          shift-right: [w141] -> _
          shift-left: dbl[] [] -> [w171]
          tunnel: ["stop"] -> w85
          tunnel: [w135] -> w84
          tunnel: w83 -> [w130]
          tunnel: w82 -> [w128]
          stop <- w134 stop-if-true
          n15 = flat-sequence {
            tunnel: w237 -> [w338]
            tunnel: w276 -> [w339]
            tunnel: w280 -> [w340]
            tunnel: w282 -> [w341]
            tunnel: w283 -> [w342]
            tunnel: w284 -> [w343]
            tunnel: w311 -> [w344]
            tunnel: w312 -> [w345]
            tunnel: w326 -> [w346]
            tunnel: w327 -> [w347]
            tunnel: w328 -> [w348]
            tunnel: [w348] -> w236
            tunnel: [w347] -> w235
            tunnel: [w346] -> w234
            tunnel: [w345] -> w233
            tunnel: [w344] -> w232
            tunnel: [w343] -> w231
            tunnel: [w342] -> w230
            tunnel: [w341] -> w229
            tunnel: [w340] -> w228
            tunnel: [w339] -> w227
            tunnel: [w338] -> w226
            tunnel: [w337] -> w208
            tunnel: [w336] -> w194
            tunnel: w193 -> [w336]
            tunnel: [w335] -> w190
            tunnel: w189 -> [w335]
            tunnel: [w334] -> w178
            tunnel: w177 -> [w334]
            tunnel: [w333] -> w176
            tunnel: w175 -> [w333]
            tunnel: [w332] -> w174
            tunnel: w173 -> [w332]
            tunnel: [w331] -> w172
            tunnel: w171 -> [w331]
            tunnel: [w330] -> w131
            tunnel: w130 -> [w330]
            tunnel: [w329] -> w129
            tunnel: w128 -> [w329]
            tunnel: [w371] -> w325
            tunnel: [w370] -> w323
            tunnel: [w366] -> w321
            tunnel: [w365] -> w316
            tunnel: [w364] -> w314
            tunnel: [w363] -> w281
            tunnel: [w362] -> w277
            tunnel: [w361] -> w257
            tunnel: [w360] -> w254
            tunnel: [w359] -> w252
            tunnel: [w358] -> w238
            tunnel: w236 -> [w371]
            tunnel: w235 -> [w370]
            tunnel: w234 -> [w369]
            tunnel: w233 -> [w365]
            tunnel: w232 -> [w364]
            tunnel: w231 -> [w361]
            tunnel: w230 -> [w360]
            tunnel: w229 -> [w359]
            tunnel: w228 -> [w363]
            tunnel: w227 -> [w362]
            tunnel: w226 -> [w358]
            tunnel: [w357] -> w209
            tunnel: w208 -> [w357]
            tunnel: w194 -> [w355]
            tunnel: [w355] -> w191
            tunnel: w190 -> [w356]
            tunnel: [w356] -> w187
            tunnel: w178 -> [w354]
            tunnel: w176 -> [w353]
            tunnel: w174 -> [w352]
            tunnel: w172 -> [w351]
            tunnel: [w354] -> w170
            tunnel: [w353] -> w166
            tunnel: [w352] -> w163
            tunnel: [w351] -> w162
            tunnel: w131 -> [w350]
            tunnel: w129 -> [w349]
            tunnel: [w350] -> w126
            tunnel: [w349] -> w124
            tunnel: w325 -> [w896]
            tunnel: [w896] -> w324
            tunnel: w323 -> [w895]
            tunnel: [w895] -> w322
            tunnel: w321 -> [w891]
            tunnel: [w891] -> w320
            tunnel: w319 -> [w892]
            tunnel: [w892] -> w318
            tunnel: [w892] -> w317
            tunnel: w316 -> [w894]
            tunnel: [w894] -> w315
            tunnel: w314 -> [w893]
            tunnel: [w893] -> w313
            tunnel: [w892] -> w310
            tunnel: [w892] -> w296
            tunnel: w281 -> [w890]
            tunnel: [w890] -> w279
            tunnel: w277 -> [w889]
            tunnel: [w889] -> w274
            tunnel: [w888] -> w258
            tunnel: w257 -> [w888]
            tunnel: [w887] -> w255
            tunnel: w254 -> [w887]
            tunnel: [w886] -> w253
            tunnel: w252 -> [w886]
            tunnel: [w885] -> w239
            tunnel: w238 -> [w885]
            tunnel: [w884] -> w210
            tunnel: w209 -> [w884]
            tunnel: [w883] -> w192
            tunnel: w191 -> [w883]
            tunnel: [w882] -> w188
            tunnel: w187 -> [w882]
            tunnel: w170 -> [w881]
            tunnel: [w881] -> w169
            tunnel: [w880] -> w167
            tunnel: w166 -> [w880]
            tunnel: [w879] -> w165
            tunnel: w163 -> [w879]
            tunnel: w162 -> [w878]
            tunnel: [w878] -> w161
            tunnel: [w877] -> w127
            tunnel: w126 -> [w877]
            tunnel: [w876] -> w125
            tunnel: w124 -> [w876]
            tunnel: [w919] -> w295
            tunnel: w324 -> [w948]
            tunnel: w322 -> [w947]
            tunnel: w320 -> [w944]
            tunnel: w318 -> [w943]
            tunnel: w317 -> [w942]
            tunnel: w315 -> [w932]
            tunnel: w313 -> [w931]
            tunnel: w310 -> [w933]
            tunnel: [w929] -> w294
            tunnel: [w930] -> w293
            tunnel: [w941] -> w292
            tunnel: [w940] -> w291
            tunnel: [w939] -> w290
            tunnel: [w938] -> w289
            tunnel: w296 -> [w928]
            tunnel: [w927] -> w288
            tunnel: [w926] -> w287
            tunnel: [w910] -> w286
            tunnel: [w925] -> w285
            tunnel: w279 -> [w924]
            tunnel: [w924] -> w278
            tunnel: [w923] -> w275
            tunnel: w274 -> [w923]
            tunnel: w258 -> [w922]
            tunnel: [w922] -> w256
            tunnel: w255 -> [w921]
            tunnel: w253 -> [w920]
            tunnel: [w921] -> w251
            tunnel: [w920] -> w250
            tunnel: w239 -> [w918]
            tunnel: [w914] -> w211
            tunnel: w210 -> [w914]
            tunnel: w192 -> [w912]
            tunnel: w188 -> [w911]
            tunnel: [w905] -> w186
            tunnel: [w910] -> w185
            tunnel: [w908] -> w184
            tunnel: [w906] -> w183
            tunnel: w169 -> [w909]
            tunnel: [w909] -> w168
            tunnel: w167 -> [w908]
            tunnel: w165 -> [w907]
            tunnel: [w907] -> w164
            tunnel: w161 -> [w906]
            tunnel: [w905] -> w139
            tunnel: [w904] -> w136
            tunnel: w127 -> [w903]
            tunnel: w125 -> [w902]
            tunnel: [w897] -> w120
            tunnel: [w898] -> w119
            tunnel: [w897] -> w118
            tunnel: [w899] -> w114
            tunnel: [w898] -> w111
            tunnel: w295 -> [w1158]
            tunnel: [w1155] -> w269
            tunnel: w294 -> [w1171]
            tunnel: [w1171] -> w268
            tunnel: w293 -> [w1170]
            tunnel: [w1170] -> w267
            tunnel: w292 -> [w1169]
            tunnel: [w1169] -> w266
            tunnel: w291 -> [w1168]
            tunnel: [w1168] -> w265
            tunnel: w290 -> [w1167]
            tunnel: [w1167] -> w264
            tunnel: w289 -> [w1166]
            tunnel: [w1166] -> w263
            tunnel: [w1159] -> w262
            tunnel: w288 -> [w1152]
            tunnel: w287 -> [w1160]
            tunnel: w286 -> [w1159]
            tunnel: w285 -> [w1161]
            tunnel: [w1158] -> w261
            tunnel: w278 -> [w1157]
            tunnel: w275 -> [w1156]
            tunnel: [w1154] -> w260
            tunnel: [w1142] -> w259
            tunnel: w256 -> [w1153]
            tunnel: w251 -> [w1150]
            tunnel: w250 -> [w1149]
            tunnel: [w1151] -> w247
            tunnel: [w1148] -> w244
            tunnel: [w1147] -> w241
            tunnel: [w1143] -> w240
            tunnel: [w1141] -> w212
            tunnel: w211 -> [w1141]
            tunnel: w186 -> [w1140]
            tunnel: w185 -> [w1139]
            tunnel: w184 -> [w1138]
            tunnel: w183 -> [w1136]
            tunnel: [w1134] -> w182
            tunnel: [w1133] -> w181
            tunnel: [w1132] -> w180
            tunnel: [w1131] -> w179
            tunnel: w168 -> [w1135]
            tunnel: w164 -> [w1137]
            tunnel: [w1134] -> w160
            tunnel: [w1133] -> w159
            tunnel: [w1132] -> w158
            tunnel: [w1131] -> w157
            tunnel: [w1130] -> w140
            tunnel: w139 -> [w1130]
            tunnel: [w1129] -> w137
            tunnel: w136 -> [w1129]
            tunnel: w120 -> [w1128]
            tunnel: w119 -> [w1127]
            tunnel: w118 -> [w1126]
            tunnel: [w1126] -> w117
            tunnel: [w1125] -> w115
            tunnel: w114 -> [w1125]
            tunnel: w111 -> [w1124]
            tunnel: [w1124] -> w110
            tunnel: w269 -> [w1205]
            tunnel: [w1212] -> w309
            tunnel: [w1211] -> w308
            tunnel: w268 -> [w1211]
            tunnel: [w1206] -> w305
            tunnel: w267 -> [w1206]
            tunnel: [w1210] -> w303
            tunnel: w266 -> [w1210]
            tunnel: [w1209] -> w301
            tunnel: w265 -> [w1209]
            tunnel: [w1208] -> w299
            tunnel: w264 -> [w1208]
            tunnel: [w1207] -> w297
            tunnel: w263 -> [w1207]
            tunnel: w262 -> [w1194]
            tunnel: w261 -> [w1195]
            tunnel: w260 -> [w1190]
            tunnel: [w1190] -> w272
            tunnel: w259 -> [w1196]
            tunnel: [w1196] -> w270
            tunnel: [w1198] -> w248
            tunnel: w247 -> [w1198]
            tunnel: [w1199] -> w245
            tunnel: w244 -> [w1199]
            tunnel: [w1200] -> w242
            tunnel: w241 -> [w1200]
            tunnel: w240 -> [w1204]
            tunnel: [w1193] -> w213
            tunnel: w212 -> [w1193]
            tunnel: w182 -> [w1189]
            tunnel: w181 -> [w1188]
            tunnel: w180 -> [w1187]
            tunnel: w179 -> [w1186]
            tunnel: w160 -> [w1185]
            tunnel: w159 -> [w1184]
            tunnel: w158 -> [w1183]
            tunnel: w157 -> [w1182]
            tunnel: [w1185] -> w155
            tunnel: [w1184] -> w153
            tunnel: [w1183] -> w151
            tunnel: [w1182] -> w149
            tunnel: w140 -> [w1181]
            tunnel: [w1180] -> w138
            tunnel: w137 -> [w1180]
            tunnel: w117 -> [w1178]
            tunnel: [w1177] -> w116
            tunnel: w115 -> [w1177]
            tunnel: w110 -> [w1176]
            tunnel: w309 -> [w1225]
            tunnel: w308 -> [w1240]
            tunnel: w305 -> [w1234]
            tunnel: w303 -> [w1239]
            tunnel: w301 -> [w1236]
            tunnel: w299 -> [w1238]
            tunnel: w297 -> [w1237]
            tunnel: w272 -> [w1230]
            tunnel: w270 -> [w1229]
            tunnel: w248 -> [w1228]
            tunnel: w245 -> [w1227]
            tunnel: w242 -> [w1226]
            tunnel: [w1219] -> w133
            tunnel: [w1240] -> w225
            tunnel: [w1234] -> w224
            tunnel: [w1239] -> w223
            tunnel: [w1236] -> w222
            tunnel: [w1238] -> w221
            tunnel: [w1237] -> w220
            tunnel: [w1230] -> w219
            tunnel: [w1229] -> w218
            tunnel: [w1228] -> w217
            tunnel: [w1227] -> w216
            tunnel: [w1226] -> w215
            tunnel: [w1224] -> w214
            tunnel: w213 -> [w1224]
            tunnel: [w1223] -> w156
            tunnel: w155 -> [w1223]
            tunnel: [w1222] -> w154
            tunnel: w153 -> [w1222]
            tunnel: [w1221] -> w152
            tunnel: w151 -> [w1221]
            tunnel: [w1220] -> w150
            tunnel: w149 -> [w1220]
            tunnel: w138 -> [w1218]
            tunnel: [w1217] -> w123
            tunnel: [w1216] -> w122
            tunnel: w116 -> [w1215]
            tunnel: [w1214] -> w113
            tunnel: [w1213] -> w112
            tunnel: w225 -> [w1286]
            tunnel: w224 -> [w1285]
            tunnel: w223 -> [w1284]
            tunnel: w222 -> [w1283]
            tunnel: w221 -> [w1282]
            tunnel: w220 -> [w1281]
            tunnel: w219 -> [w1280]
            tunnel: w218 -> [w1279]
            tunnel: w217 -> [w1278]
            tunnel: w216 -> [w1277]
            tunnel: w215 -> [w1276]
            tunnel: w214 -> [w1271]
            tunnel: [w1286] -> w207
            tunnel: [w1285] -> w206
            tunnel: [w1284] -> w205
            tunnel: [w1283] -> w204
            tunnel: [w1282] -> w203
            tunnel: [w1281] -> w202
            tunnel: [w1280] -> w201
            tunnel: [w1279] -> w200
            tunnel: [w1278] -> w199
            tunnel: [w1277] -> w198
            tunnel: [w1276] -> w197
            tunnel: [w1271] -> w196
            tunnel: [w1270] -> w195
            tunnel: w156 -> [w1269]
            tunnel: w154 -> [w1268]
            tunnel: w152 -> [w1267]
            tunnel: w150 -> [w1266]
            tunnel: [w1269] -> w148
            tunnel: [w1268] -> w146
            tunnel: [w1267] -> w144
            tunnel: [w1266] -> w142
            tunnel: w123 -> [w1265]
            tunnel: w122 -> [w1264]
            tunnel: [w1259] -> w121
            tunnel: w113 -> [w1258]
            tunnel: w112 -> [w1257]
            tunnel: [w1297] -> w243
            tunnel: [w1298] -> w246
            tunnel: [w1299] -> w249
            tunnel: [w1300] -> w271
            tunnel: [w1301] -> w273
            tunnel: [w1302] -> w298
            tunnel: [w1303] -> w300
            tunnel: [w1304] -> w302
            tunnel: [w1305] -> w304
            tunnel: [w1306] -> w306
            tunnel: [w1307] -> w307
            tunnel: w207 -> [w1307]
            tunnel: w206 -> [w1306]
            tunnel: w205 -> [w1305]
            tunnel: w204 -> [w1304]
            tunnel: w203 -> [w1303]
            tunnel: w202 -> [w1302]
            tunnel: w201 -> [w1301]
            tunnel: w200 -> [w1300]
            tunnel: w199 -> [w1299]
            tunnel: w198 -> [w1298]
            tunnel: w197 -> [w1297]
            tunnel: w196 -> [w1293]
            tunnel: w195 -> [w1292]
            tunnel: [w1291] -> w147
            tunnel: w148 -> [w1291]
            tunnel: [w1290] -> w145
            tunnel: w146 -> [w1290]
            tunnel: [w1289] -> w143
            tunnel: w144 -> [w1289]
            tunnel: [w1288] -> w141
            tunnel: w142 -> [w1288]
            tunnel: [w1287] -> w135
            tunnel: w121 -> [w1287]
            frame #0 {
              n16 = Tick Count (ms)() -> (millisecond timer value=w337:u32)
            }
            frame #1 {
              n17 = while {
                tunnel: w369 -> [w376]
                tunnel: [w375] -> w368
                tunnel: [w374] -> w367
                tunnel: w355 -> [w372]
                stop <- w377 stop-if-true
                n18 = event shown="[0] Timeout" {
                  selector: _ -> [_ _ _ _ _ _ _ _ _ _ _ _]
                  dyn-events: _ -> [_ _ _ _ _ _ _ _ _ _ _ _]
                  timeout: 1 -> [_ _ _ _ _ _ _ _ _ _ _ _]
                  tunnel: [TRUE ("Set Gauge to Zero") w385 w434 w455 w481 w516 w572 w623 w702 w773 "Set Gauge to Zero" _] -> w377
                  tunnel: w376 -> [w381 w384 w431 w453 w477 w515 w568 w621 w700 w771 w848 w870]
                  tunnel: [w380 w383 w430 w452 w479 w513 w570 w620 w699 w770 w847 w869] -> w375
                  tunnel: [w379 w382 w429 w451 w478 w514 w569 w619 w698 w769 w846 w868] -> w374
                  tunnel: w372 -> [_ _ _ _ _ _ _ _ _ _ w844 _]
                  event Timeout {
                    n19 = event-data() -> ()  [unwired: 1 in, 1 out]
                    n20 = Unbundle(w381) -> ("VISA resource name out"=w380:refnum<visa-resource-name>, "error out"=w379:errorcluster)  [unwired: 2 out]
                  }
                  event "Setpoint\n START": Value Change {
                    n21 = event-data() -> ()  [unwired: 1 in, 1 out]
                    n22 = stacked-sequence {
                      tunnel: w384 -> [_ w391 _]
                      tunnel: [_ w390 _] -> w382
                      tunnel: [_ w389 _] -> w383
                      frame #0 {
                        n23 = property on="Setpoint\n START" class="Bool"("Blinking"=TRUE) -> ()  [unwired: 2 in, 2 out]
                        n24 = property on="ON" class="Bool (strict)"("Blinking"=FALSE) -> ()  [unwired: 2 in, 2 out]
                      }
                      frame #1 {
                        n25 = for {
                          N: 2 -> [_]
                          tunnel: w391 -> [w395]
                          tunnel: [w394] -> w390
                          tunnel: [w393] -> w389
                          i -> [w397]
                          n26 = flat-sequence {
                            tunnel: [w400] -> w396
                            tunnel: w397 -> [w399]
                            tunnel: [w418] -> w398
                            tunnel: w396 -> [w417]
                            tunnel: w395 -> [w419]
                            tunnel: [w416] -> w394
                            tunnel: [w415] -> w393
                            tunnel: w398 -> [w425]
                            tunnel: w397 -> [w424]
                            frame #0 {
                              n27 = case shown="0, Default" w399 {
                                tunnel: [w409 w411] -> w400
                                frame 0, Default {
                                n28 = Multiply(x=10.0, y="SP 1 input (°C)") -> (x*y=w406:dbl)
                                n29 = local read "RAM"() -> (w404:bool)
                                n30 = Number To Hexadecimal String(1:i16 5 ("width (-)"), 2:w406) -> (0:w408:string)
                                n31 = Select(t="*P012", s=w404, f="*P012") -> (s? t:f=w401:string)
                                n32 = Concatenate Strings(w401, w408) -> (w409:string)
                                }
                                frame 1 {
                                n33 = local read "RAM"() -> (w414:bool)
                                n34 = Select(t="*G01", s=w414, f="*R01") -> (s? t:f=w411:string)
                                }
                              }
                            }
                            frame #1 {
                              n35 = Unbundle(w419) -> ("VISA resource name out"=w420:refnum<visa-resource-name>, "error out"=w422:errorcluster, "Delay (ms)"=w421:u32, "Write/\nRead"=w423:bool)
                              n36 = call "I3252_Comm_Interface.vi"("VISA resource name in"=w420, "error in"=w422, "Delay (ms)"=w421, "Write"=w423, "String to Write"=w417, "Read"=w423) -> ("VISA resource name out"=w415:refnum<visa-resource-name>, "error out"=w416:errorcluster, "Read String"=w418:string)  [unwired: 2 in]
                            }
                            frame #2 {
                              n37 = case shown="0, Default" w424 {
                                tunnel: w425 -> [_ w427]
                                frame 0, Default {
                                }
                                frame 1 {
                                n38 = call "I3252_Edit_Setpoint.vi"("Read String"=w427) -> ("Setpoint is"=→"SP 1 is (°C)":dbl)
                                }
                              }
                            }
                          }
                        }
                      }
                      frame #2 {
                        n39 = property on="Setpoint\n START" class="Bool"("Blinking"=FALSE) -> ()  [unwired: 2 in, 2 out]
                      }
                    }
                    n40 = Not(x="Setpoint\n START") -> (.not. x?=w385:bool)
                  }
                  event "Standby": Value Change {
                    n41 = event-data() -> ()  [unwired: 1 in, 1 out]
                    n42 = flat-sequence {
                      tunnel: [w442] -> w432
                      tunnel: w432 -> [w446]
                      tunnel: w431 -> [w445]
                      tunnel: [w444] -> w429
                      tunnel: [w443] -> w430
                      frame #0 {
                        n43 = local read "Standby"() -> (w435:bool)
                        n44 = Select(t=TRUE, s=w435, f=FALSE) -> (s? t:f=w438:bool)
                        n45 = property on="Standby" class="Bool (strict)"("Blinking"=w438) -> ()  [unwired: 2 in, 2 out]
                      }
                      frame #1 {
                        n46 = local read "Standby"() -> (w440:bool)
                        n47 = Select(t="*D03", s=w440, f="*E03") -> (s? t:f=w442:string)
                      }
                      frame #2 {
                        n48 = Unbundle(w445) -> ("VISA resource name out"=w447:refnum<visa-resource-name>, "error out"=w449:errorcluster, "Delay (ms)"=w448:u32, "Write/\nRead"=w450:bool)
                        n49 = call "I3252_Comm_Interface.vi"("VISA resource name in"=w447, "error in"=w449, "Delay (ms)"=w448, "Write"=w450, "String to Write"=w446, "Read"=w450) -> ("VISA resource name out"=w443:refnum<visa-resource-name>, "error out"=w444:errorcluster)  [unwired: 2 in, 1 out]
                      }
                    }
                    n50 = Not(x="Standby") -> (.not. x?=w434:bool)
                  }
                  event "Set Command": Value Change {
                    n51 = event-data() -> ()  [unwired: 1 in, 1 out]
                    n52 = stacked-sequence {
                      tunnel: w453 -> [_ w460 _]
                      tunnel: [_ w459 _] -> w452
                      tunnel: [_ w458 _] -> w451
                      frame #0 {
                        n53 = property on="Set Command" class="Bool"("Blinking"=TRUE) -> ()  [unwired: 2 in, 2 out]
                        n54 = property on="ON" class="Bool (strict)"("Blinking"=FALSE) -> ()  [unwired: 2 in, 2 out]
                      }
                      frame #1 {
                        n55 = flat-sequence {
                          tunnel: [w465] -> w462
                          tunnel: [w468] -> w461
                          tunnel: w462 -> [w469]
                          tunnel: w460 -> [w470]
                          tunnel: [w467] -> w459
                          tunnel: [w466] -> _
                          tunnel: [w466] -> w458
                          tunnel: w461 -> [w475]
                          frame #0 {
                            n56 = Concatenate Strings("*", "Command input") -> (w465:string)
                          }
                          frame #1 {
                            n57 = Unbundle(w470) -> ("VISA resource name out"=w474:refnum<visa-resource-name>, "error out"=w472:errorcluster, "Delay (ms)"=w473:u32, "Write/\nRead"=w471:bool)
                            n58 = call "I3252_Comm_Interface.vi"("VISA resource name in"=w474, "error in"=w472, "Delay (ms)"=w473, "Write"=w471, "String to Write"=w469, "Read"=w471) -> ("VISA resource name out"=w467:refnum<visa-resource-name>, "error out"=w466:errorcluster, "Read String"=w468:string)  [unwired: 2 in]
                          }
                          frame #2 {
                            "Command output" <- w475
                          }
                        }
                      }
                      frame #2 {
                        n59 = property on="Set Command" class="Bool"("Blinking"=FALSE) -> ()  [unwired: 2 in, 2 out]
                      }
                    }
                    n60 = Not(x="Set Command") -> (.not. x?=w455:bool)
                  }
                  event "Reset\nSTOPP": Value Change {
                    n61 = event-data() -> ()  [unwired: 1 in, 1 out]
                    n62 = stacked-sequence {
                      tunnel: [_ w488 _] -> w478
                      tunnel: [_ w487 _] -> w479
                      tunnel: w477 -> [_ w485 _]
                      frame #0 {
                        n63 = property on="Reset\nSTOPP" class="Bool"("Blinking"=TRUE) -> ()  [unwired: 2 in, 2 out]
                        n64 = property on="ON" class="Bool (strict)"("Blinking"=FALSE) -> ()  [unwired: 2 in, 2 out]
                      }
                      frame #1 {
                        n65 = for {
                          N: 2 -> [_]
                          tunnel: [w494] -> w488
                          tunnel: [w493] -> w487
                          tunnel: w485 -> [w492]
                          i -> [w490]
                          n66 = flat-sequence {
                            tunnel: w490 -> [w496]
                            tunnel: [w495] -> w491
                            tunnel: [w501] -> w494
                            tunnel: [w502] -> w493
                            tunnel: w492 -> [w503]
                            tunnel: w491 -> [w500]
                            tunnel: [w499] -> w489
                            tunnel: w490 -> [w509]
                            tunnel: w489 -> [w508]
                            frame #0 {
                              n67 = case shown="0, Default" w496 {
                                tunnel: ["*Z02" "*G01"] -> w495
                                frame 0, Default {
                                }
                                frame 1 {
                                }
                              }
                            }
                            frame #1 {
                              n68 = Unbundle(w503) -> ("VISA resource name out"=w504:refnum<visa-resource-name>, "error out"=w506:errorcluster, "Delay (ms)"=w505:u32, "Write/\nRead"=w507:bool)
                              n69 = call "I3252_Comm_Interface.vi"("VISA resource name in"=w504, "error in"=w506, "Delay (ms)"=w505, "Write"=w507, "String to Write"=w500, "Read"=w507) -> ("VISA resource name out"=w502:refnum<visa-resource-name>, "error out"=w501:errorcluster, "Read String"=w499:string)  [unwired: 2 in]
                            }
                            frame #2 {
                              n70 = case shown="0, Default" w509 {
                                tunnel: w508 -> [_ w511]
                                frame 0, Default {
                                }
                                frame 1 {
                                n71 = call "I3252_Edit_Setpoint.vi"("Read String"=w511) -> ("Setpoint is"=w510:dbl)
                                n72 = local write "SP 1 is (°C)"(w510) -> ()
                                }
                              }
                            }
                          }
                        }
                        n73 = Wait (ms)(milliseconds to wait=u32 4000) -> ()  [unwired: 1 out]
                      }
                      frame #2 {
                        n74 = property on="Reset\nSTOPP" class="Bool"("Blinking"=FALSE) -> ()  [unwired: 2 in, 2 out]
                      }
                    }
                    n75 = Not(x="Reset\nSTOPP") -> (.not. x?=w481:bool)
                  }
                  event "Auto Tune": Value Change {
                    n76 = event-data() -> ()  [unwired: 1 in, 1 out]
                    n77 = stacked-sequence {
                      tunnel: w515 -> [_ w522 w567]
                      tunnel: [_ w521 _] -> w514
                      tunnel: [_ w520 _] -> w513
                      frame #0 {
                        n78 = property on="Auto Tune" class="Bool"("Blinking"=TRUE) -> ()  [unwired: 2 in, 2 out]
                        n79 = property on="ON" class="Bool (strict)"("Blinking"=FALSE) -> ()  [unwired: 2 in, 2 out]
                      }
                      frame #1 {
                        n80 = for {
                          N: 4 -> [_]
                          tunnel: [w527] -> w520
                          tunnel: [w526] -> w521
                          tunnel: w522 -> [w525]
                          i -> [w530]
                          n81 = flat-sequence {
                            tunnel: w530 -> [w532]
                            tunnel: [w531] -> w528
                            tunnel: w528 -> [w547]
                            tunnel: [w546] -> w529
                            tunnel: [w549] -> w527
                            tunnel: [w548] -> w526
                            tunnel: w525 -> [w545]
                            tunnel: w530 -> [w555]
                            tunnel: w529 -> [w554]
                            frame #0 {
                              n82 = case shown="0, Default" w532 {
                                tunnel: ["*V01" w535 "*W0C35" "*Z02"] -> w531
                                frame 0, Default {
                                }
                                frame 1 {
                                n83 = local read "(°C)"() -> (w534:dbl)
                                n84 = Add(x=20.0, y=w534) -> (x+y=w541:dbl)
                                n85 = Multiply(x=10.0, y=w541) -> (x*y=w538:dbl)
                                n86 = Number To Hexadecimal String(1:i16 5 ("width (-)"), 2:w538) -> (0:w537:string)
                                n87 = Concatenate Strings("*W012", w537) -> (w535:string)
                                }
                                frame 2 {
                                # "35 hex = \n00110101 bin"
                                }
                                frame 3 {
                                }
                              }
                            }
                            frame #1 {
                              n88 = Unbundle(w545) -> ("VISA resource name out"=w553:refnum<visa-resource-name>, "error out"=w551:errorcluster, "Delay (ms)"=w552:u32, "Write/\nRead"=w550:bool)
                              n89 = call "I3252_Comm_Interface.vi"("VISA resource name in"=w553, "error in"=w551, "Delay (ms)"=w552, "Write"=w550, "String to Write"=w547, "Read"=w550) -> ("VISA resource name out"=w549:refnum<visa-resource-name>, "error out"=w548:errorcluster, "Read String"=w546:string)  [unwired: 2 in]
                            }
                            frame #2 {
                              n90 = case shown="0, Default" w555 {
                                tunnel: w554 -> [w557]
                                frame 0, Default {
                                n91 = call <vilib>:"Space Constant.vi"() -> ("String"=w560:string)
                                n92 = Search/Split String(string=w557, search string/char (-)=w560) -> (match + rest of string=w559:string)  [unwired: 1 in, 2 out]
                                n93 = Fract/Exp String To Number(use system decimal point (T)=FALSE, string=w559) -> (number=w556:dbl)  [unwired: 2 in, 1 out]
                                n94 = local write "(°C)"(w556) -> ()
                                }
                              }
                            }
                          }
                        }
                        n95 = Wait (ms)(milliseconds to wait=u32 45000) -> ()  [unwired: 1 out]
                      }
                      frame #2 {
                        n96 = Unbundle(w567) -> ("VISA resource name out"=w566:refnum<visa-resource-name>, "error out"=w564:errorcluster, "Delay (ms)"=w565:u32, "Write/\nRead"=w563:bool)
                        n97 = property on="Auto Tune" class="Bool"("Blinking"=FALSE) -> ()  [unwired: 2 in, 2 out]
                        n98 = call "I3252_Comm_Interface.vi"("VISA resource name in"=w566, "error in"=w564, "Delay (ms)"=w565, "Write"=w563, "String to Write"="*W01200000", "Read"=w563) -> ()  [unwired: 2 in, 3 out]
                      }
                    }
                    n99 = Not(x="Auto Tune") -> (.not. x?=w516:bool)
                  }
                  event "Write LOW/HI": Value Change {
                    n100 = event-data() -> ()  [unwired: 1 in, 1 out]
                    n101 = stacked-sequence {
                      tunnel: [_ w577 _] -> w570
                      tunnel: [_ w576 _] -> w569
                      tunnel: w568 -> [_ w575 _]
                      frame #0 {
                        n102 = property on="Write LOW/HI" class="Bool"("Blinking"=TRUE) -> ()  [unwired: 2 in, 2 out]
                        n103 = property on="ON" class="Bool (strict)"("Blinking"=FALSE) -> ()  [unwired: 2 in, 2 out]
                      }
                      frame #1 {
                        n104 = for {
                          N: 4 -> [_]
                          tunnel: [w581] -> w577
                          tunnel: [w580] -> w576
                          tunnel: w575 -> [w579]
                          i -> [w583]
                          n105 = flat-sequence {
                            tunnel: w583 -> [w585]
                            tunnel: [w586] -> w582
                            tunnel: w582 -> [w600]
                            tunnel: [w601] -> w584
                            tunnel: [w603] -> w581
                            tunnel: [w602] -> w580
                            tunnel: w579 -> [w599]
                            tunnel: w584 -> [w609]
                            tunnel: w583 -> [w608]
                            frame #0 {
                              n106 = case shown="1" w585 {
                                tunnel: [w588 w594 "*R27" "*R28"] -> w586
                                frame 0, Default {
                                n107 = Number To Hexadecimal String(1:i16 2 ("width (-)"), 2:"% LOW Sollwert") -> (0:w589:string)
                                n108 = Concatenate Strings("*W27", w589) -> (w588:string)
                                }
                                frame 1 {
                                n109 = Number To Hexadecimal String(1:i16 2 ("width (-)"), 2:"% High Sollwert") -> (0:w595:string)
                                n110 = Concatenate Strings("*W28", w595) -> (w594:string)
                                }
                                frame 2 {
                                }
                                frame 3 {
                                }
                              }
                            }
                            frame #1 {
                              n111 = Unbundle(w599) -> ("VISA resource name out"=w607:refnum<visa-resource-name>, "error out"=w605:errorcluster, "Delay (ms)"=w606:u32, "Write/\nRead"=w604:bool)
                              n112 = call "I3252_Comm_Interface.vi"("VISA resource name in"=w607, "error in"=w605, "Delay (ms)"=w606, "Write"=w604, "String to Write"=w600, "Read"=w604) -> ("VISA resource name out"=w603:refnum<visa-resource-name>, "error out"=w602:errorcluster, "Read String"=w601:string)  [unwired: 2 in]
                            }
                            frame #2 {
                              n113 = case shown="0, Default" w608 {
                                tunnel: w609 -> [_ w613 w617]
                                frame 0, Default {
                                }
                                frame 2 {
                                n114 = String Subset(string=w613, offset (0)=3) -> (substring=w611:string)  [unwired: 1 in]
                                n115 = Hexadecimal String To Number(string=w611) -> (number=→"% LOW Istwert":u32)  [unwired: 2 in, 1 out]
                                }
                                frame 3 {
                                n116 = String Subset(string=w617, offset (0)=3) -> (substring=w615:string)  [unwired: 1 in]
                                n117 = Hexadecimal String To Number(string=w615) -> (number=→"% HIGH Istwert":u32)  [unwired: 2 in, 1 out]
                                }
                              }
                            }
                          }
                        }
                      }
                      frame #2 {
                        n118 = property on="Write LOW/HI" class="Bool"("Blinking"=FALSE) -> ()  [unwired: 2 in, 2 out]
                      }
                    }
                    n119 = Not(x="Write LOW/HI") -> (.not. x?=w572:bool)
                  }
                  event "Set PID": Value Change {
                    n120 = event-data() -> ()  [unwired: 1 in, 1 out]
                    n121 = stacked-sequence {
                      tunnel: w621 -> [_ w628 _]
                      tunnel: [_ w627 _] -> w620
                      tunnel: [_ w626 _] -> w619
                      frame #0 {
                        n122 = property on="Set PID" class="Bool"("Blinking"=TRUE) -> ()  [unwired: 2 in, 2 out]
                        n123 = property on="ON" class="Bool (strict)"("Blinking"=FALSE) -> ()  [unwired: 2 in, 2 out]
                      }
                      frame #1 {
                        n124 = for {
                          N: 6 -> [_]
                          tunnel: w628 -> [w632]
                          tunnel: [w631] -> w627
                          tunnel: [w630] -> w626
                          i -> [w634]
                          n125 = flat-sequence {
                            tunnel: w634 -> [w636]
                            tunnel: [w637] -> w633
                            tunnel: w633 -> [w678]
                            tunnel: [w674] -> w635
                            tunnel: w632 -> [w677]
                            tunnel: [w676] -> w630
                            tunnel: [w675] -> w631
                            tunnel: w635 -> [w684]
                            tunnel: w634 -> [w683]
                            frame #0 {
                              n126 = case shown="0, Default" w636 {
                                tunnel: [w644 w652 w660 w662 w666 w670] -> w637
                                frame 0, Default {
                                n127 = local read "RAM"() -> (w638:bool)
                                n128 = Number To Hexadecimal String(1:i16 4 ("width (-)"), 2:"P (PB1) Sollwert") -> (0:w645:string)
                                n129 = Select(t="*P17", s=w638, f="*W17") -> (s? t:f=w639:string)
                                n130 = Concatenate Strings(w639, w645) -> (w644:string)
                                }
                                frame 1 {
                                n131 = local read "RAM"() -> (w646:bool)
                                n132 = Number To Hexadecimal String(1:i16 4 ("width (-)"), 2:"I ( Reset1) Sollwert") -> (0:w653:string)
                                n133 = Select(t="*P18", s=w646, f="*W18") -> (s? t:f=w648:string)
                                n134 = Concatenate Strings(w648, w653) -> (w652:string)
                                }
                                frame 2 {
                                n135 = local read "RAM"() -> (w655:bool)
                                n136 = Number To Hexadecimal String(1:i16 4 ("width (-)"), 2:"D (Rate) Sollwert") -> (0:w661:string)
                                n137 = Select(t="*P19", s=w655, f="*W19") -> (s? t:f=w656:string)
                                n138 = Concatenate Strings(w656, w661) -> (w660:string)
                                }
                                frame 3 {
                                n139 = local read "RAM"() -> (w665:bool)
                                n140 = Select(t="*G17", s=w665, f="*R17") -> (s? t:f=w662:string)
                                }
                                frame 4 {
                                n141 = local read "RAM"() -> (w669:bool)
                                n142 = Select(t="*G18", s=w669, f="*R18") -> (s? t:f=w666:string)
                                }
                                frame 5 {
                                n143 = local read "RAM"() -> (w673:bool)
                                n144 = Select(t="*G19", s=w673, f="*R19") -> (s? t:f=w670:string)
                                }
                              }
                            }
                            frame #1 {
                              n145 = Unbundle(w677) -> ("VISA resource name out"=w682:refnum<visa-resource-name>, "error out"=w680:errorcluster, "Delay (ms)"=w681:u32, "Write/\nRead"=w679:bool)
                              n146 = call "I3252_Comm_Interface.vi"("VISA resource name in"=w682, "error in"=w680, "Delay (ms)"=w681, "Write"=w679, "String to Write"=w678, "Read"=w679) -> ("VISA resource name out"=w675:refnum<visa-resource-name>, "error out"=w676:errorcluster, "Read String"=w674:string)  [unwired: 2 in]
                            }
                            frame #2 {
                              n147 = case shown="5" w683 {
                                tunnel: w684 -> [_ w688 w692 w696]
                                frame 0, Default {
                                }
                                frame 3 {
                                n148 = String Subset(string=w688, offset (0)=3) -> (substring=w686:string)  [unwired: 1 in]
                                n149 = Hexadecimal String To Number(string=w686) -> (number=→"P (PB1) Istwert":u32)  [unwired: 2 in, 1 out]
                                }
                                frame 4 {
                                n150 = String Subset(string=w692, offset (0)=3) -> (substring=w690:string)  [unwired: 1 in]
                                n151 = Hexadecimal String To Number(string=w690) -> (number=→"I ( Reset1) Istwert":u32)  [unwired: 2 in, 1 out]
                                }
                                frame 5 {
                                n152 = String Subset(string=w696, offset (0)=3) -> (substring=w694:string)  [unwired: 1 in]
                                n153 = Hexadecimal String To Number(string=w694) -> (number=→"D (Rate) IstWert":u32)  [unwired: 2 in, 1 out]
                                }
                              }
                            }
                          }
                        }
                      }
                      frame #2 {
                        n154 = property on="Set PID" class="Bool"("Blinking"=FALSE) -> ()  [unwired: 2 in, 2 out]
                      }
                    }
                    n155 = Not(x="Set PID") -> (.not. x?=w623:bool)
                  }
                  event "Get Values": Value Change {
                    n156 = event-data() -> ()  [unwired: 1 in, 1 out]
                    n157 = stacked-sequence {
                      tunnel: w700 -> [_ w707 _]
                      tunnel: [_ w706 _] -> w699
                      tunnel: [_ w705 _] -> w698
                      frame #0 {
                        n158 = property on="Get Values" class="Bool"("Blinking"=TRUE) -> ()  [unwired: 2 in, 2 out]
                        n159 = property on="ON" class="Bool (strict)"("Blinking"=FALSE) -> ()  [unwired: 2 in, 2 out]
                      }
                      frame #1 {
                        n160 = for {
                          N: 6 -> [_]
                          tunnel: w707 -> [w711]
                          tunnel: [w710] -> w706
                          tunnel: [w709] -> w705
                          i -> [w713]
                          n161 = flat-sequence {
                            tunnel: w713 -> [w715]
                            tunnel: [w716] -> w712
                            tunnel: w712 -> [w738]
                            tunnel: [w739] -> w714
                            tunnel: w711 -> [w737]
                            tunnel: [w736] -> w709
                            tunnel: [w735] -> w710
                            tunnel: w714 -> [w745]
                            tunnel: w713 -> [w744]
                            frame #0 {
                              n162 = case shown="0, Default" w715 {
                                tunnel: [w719 w723 w727 "*R27" "*R28" w733] -> w716
                                frame 0, Default {
                                n163 = local read "RAM"() -> (w720:bool)
                                n164 = Select(t="*G17", s=w720, f="*R17") -> (s? t:f=w719:string)
                                }
                                frame 1 {
                                n165 = local read "RAM"() -> (w724:bool)
                                n166 = Select(t="*G18", s=w724, f="*R18") -> (s? t:f=w723:string)
                                }
                                frame 2 {
                                n167 = local read "RAM"() -> (w728:bool)
                                n168 = Select(t="*G19", s=w728, f="*R19") -> (s? t:f=w727:string)
                                }
                                frame 3 {
                                }
                                frame 4 {
                                }
                                frame 5 {
                                n169 = local read "RAM"() -> (w734:bool)
                                n170 = Select(t="*G01", s=w734, f="*R01") -> (s? t:f=w733:string)
                                }
                              }
                            }
                            frame #1 {
                              n171 = Unbundle(w737) -> ("VISA resource name out"=w743:refnum<visa-resource-name>, "error out"=w741:errorcluster, "Delay (ms)"=w742:u32, "Write/\nRead"=w740:bool)
                              n172 = call "I3252_Comm_Interface.vi"("VISA resource name in"=w743, "error in"=w741, "Delay (ms)"=w742, "Write"=w740, "String to Write"=w738, "Read"=w740) -> ("VISA resource name out"=w735:refnum<visa-resource-name>, "error out"=w736:errorcluster, "Read String"=w739:string)  [unwired: 2 in]
                            }
                            frame #2 {
                              n173 = case shown="0, Default" w744 {
                                tunnel: w745 -> [w747 w751 w755 w759 w763 w767]
                                frame 0, Default {
                                n174 = String Subset(string=w747, offset (0)=3) -> (substring=w748:string)  [unwired: 1 in]
                                n175 = Hexadecimal String To Number(string=w748) -> (number=w746:u32)  [unwired: 2 in, 1 out]
                                n176 = local write "P (PB1) Sollwert"(w746) -> ()
                                n177 = local write "P (PB1) Istwert"(w746) -> ()
                                }
                                frame 1 {
                                n178 = String Subset(string=w751, offset (0)=3) -> (substring=w752:string)  [unwired: 1 in]
                                n179 = Hexadecimal String To Number(string=w752) -> (number=w750:u32)  [unwired: 2 in, 1 out]
                                n180 = local write "I ( Reset1) Sollwert"(w750) -> ()
                                n181 = local write "I ( Reset1) Istwert"(w750) -> ()
                                }
                                frame 2 {
                                n182 = String Subset(string=w755, offset (0)=3) -> (substring=w756:string)  [unwired: 1 in]
                                n183 = Hexadecimal String To Number(string=w756) -> (number=w754:u32)  [unwired: 2 in, 1 out]
                                n184 = local write "D (Rate) Sollwert"(w754) -> ()
                                n185 = local write "D (Rate) IstWert"(w754) -> ()
                                }
                                frame 3 {
                                n186 = String Subset(string=w759, offset (0)=3) -> (substring=w760:string)  [unwired: 1 in]
                                n187 = Hexadecimal String To Number(string=w760) -> (number=w758:u32)  [unwired: 2 in, 1 out]
                                n188 = local write "% LOW Istwert"(w758) -> ()
                                n189 = local write "% LOW Sollwert"(w758) -> ()
                                }
                                frame 4 {
                                n190 = String Subset(string=w763, offset (0)=3) -> (substring=w764:string)  [unwired: 1 in]
                                n191 = Hexadecimal String To Number(string=w764) -> (number=w762:u32)  [unwired: 2 in, 1 out]
                                n192 = local write "% High Sollwert"(w762) -> ()
                                n193 = local write "% HIGH Istwert"(w762) -> ()
                                }
                                frame 5 {
                                n194 = call "I3252_Edit_Setpoint.vi"("Read String"=w767) -> ("Setpoint is"=w766:dbl)
                                n195 = local write "SP 1 is (°C)"(w766) -> ()
                                }
                              }
                            }
                          }
                        }
                      }
                      frame #2 {
                        n196 = property on="Get Values" class="Bool"("Blinking"=FALSE) -> ()  [unwired: 2 in, 2 out]
                      }
                    }
                    n197 = Not(x="Get Values") -> (.not. x?=w702:bool)
                  }
                  event "RAM": Value Change {
                    n198 = event-data() -> ()  [unwired: 1 in, 1 out]
                    n199 = stacked-sequence {
                      tunnel: w771 -> [_ w778 _]
                      tunnel: [_ w777 _] -> w770
                      tunnel: [_ w776 _] -> w769
                      frame #0 {
                        n200 = property on="RAM" class="Bool (strict)"("Blinking"=TRUE) -> ()  [unwired: 2 in, 2 out]
                        n201 = property on="ON" class="Bool (strict)"("Blinking"=FALSE) -> ()  [unwired: 2 in, 2 out]
                      }
                      frame #1 {
                        n202 = for {
                          N: 6 -> [_]
                          tunnel: w778 -> [w782]
                          tunnel: [w781] -> w777
                          tunnel: [w780] -> w776
                          i -> [w784]
                          n203 = flat-sequence {
                            tunnel: w784 -> [w786]
                            tunnel: [w787] -> w783
                            tunnel: w783 -> [w806]
                            tunnel: [w807] -> w785
                            tunnel: w782 -> [w810]
                            tunnel: [w809] -> w780
                            tunnel: [w808] -> w781
                            tunnel: w785 -> [w816]
                            tunnel: w784 -> [w815]
                            frame #0 {
                              n204 = case shown="0, Default" w786 {
                                tunnel: [w790 w794 w798 "*R27" "*R28" w804] -> w787
                                frame 0, Default {
                                n205 = local read "RAM"() -> (w791:bool)
                                n206 = Select(t="*G17", s=w791, f="*R17") -> (s? t:f=w790:string)
                                }
                                frame 1 {
                                n207 = local read "RAM"() -> (w795:bool)
                                n208 = Select(t="*G18", s=w795, f="*R18") -> (s? t:f=w794:string)
                                }
                                frame 2 {
                                n209 = local read "RAM"() -> (w799:bool)
                                n210 = Select(t="*G19", s=w799, f="*R19") -> (s? t:f=w798:string)
                                }
                                frame 3 {
                                }
                                frame 4 {
                                }
                                frame 5 {
                                n211 = local read "RAM"() -> (w805:bool)
                                n212 = Select(t="*G01", s=w805, f="*R01") -> (s? t:f=w804:string)
                                }
                              }
                            }
                            frame #1 {
                              n213 = Unbundle(w810) -> ("VISA resource name out"=w814:refnum<visa-resource-name>, "error out"=w812:errorcluster, "Delay (ms)"=w813:u32, "Write/\nRead"=w811:bool)
                              n214 = call "I3252_Comm_Interface.vi"("VISA resource name in"=w814, "error in"=w812, "Delay (ms)"=w813, "Write"=w811, "String to Write"=w806, "Read"=w811) -> ("VISA resource name out"=w808:refnum<visa-resource-name>, "error out"=w809:errorcluster, "Read String"=w807:string)  [unwired: 2 in]
                            }
                            frame #2 {
                              n215 = case shown="0, Default" w815 {
                                tunnel: w816 -> [w818 w822 w826 w830 w834 w838]
                                frame 0, Default {
                                n216 = String Subset(string=w818, offset (0)=3) -> (substring=w819:string)  [unwired: 1 in]
                                n217 = Hexadecimal String To Number(string=w819) -> (number=w817:u32)  [unwired: 2 in, 1 out]
                                n218 = local write "P (PB1) Sollwert"(w817) -> ()
                                n219 = local write "P (PB1) Istwert"(w817) -> ()
                                }
                                frame 1 {
                                n220 = String Subset(string=w822, offset (0)=3) -> (substring=w823:string)  [unwired: 1 in]
                                n221 = Hexadecimal String To Number(string=w823) -> (number=w821:u32)  [unwired: 2 in, 1 out]
                                n222 = local write "I ( Reset1) Sollwert"(w821) -> ()
                                n223 = local write "I ( Reset1) Istwert"(w821) -> ()
                                }
                                frame 2 {
                                n224 = String Subset(string=w826, offset (0)=3) -> (substring=w827:string)  [unwired: 1 in]
                                n225 = Hexadecimal String To Number(string=w827) -> (number=w825:u32)  [unwired: 2 in, 1 out]
                                n226 = local write "D (Rate) IstWert"(w825) -> ()
                                n227 = local write "D (Rate) Sollwert"(w825) -> ()
                                }
                                frame 3 {
                                n228 = String Subset(string=w830, offset (0)=3) -> (substring=w831:string)  [unwired: 1 in]
                                n229 = Hexadecimal String To Number(string=w831) -> (number=w829:u32)  [unwired: 2 in, 1 out]
                                n230 = local write "% LOW Istwert"(w829) -> ()
                                n231 = local write "% LOW Sollwert"(w829) -> ()
                                }
                                frame 4 {
                                n232 = String Subset(string=w834, offset (0)=3) -> (substring=w835:string)  [unwired: 1 in]
                                n233 = Hexadecimal String To Number(string=w835) -> (number=w833:u32)  [unwired: 2 in, 1 out]
                                n234 = local write "% HIGH Istwert"(w833) -> ()
                                n235 = local write "% High Sollwert"(w833) -> ()
                                }
                                frame 5 {
                                n236 = call "I3252_Edit_Setpoint.vi"("Read String"=w838) -> ("Setpoint is"=w837:dbl)
                                n237 = local write "SP 1 is (°C)"(w837) -> ()
                                }
                              }
                            }
                          }
                        }
                      }
                      frame #2 {
                        n238 = property on="RAM" class="Bool (strict)"("Blinking"=FALSE) -> ()  [unwired: 2 in, 2 out]
                      }
                    }
                    n239 = Not(x="RAM") -> (.not. x?=w773:bool)
                  }
                  event "Set Gauge to Zero": Value Change {
                    n240 = event-data() -> ()  [unwired: 1 in, 1 out]
                    n241 = flat-sequence {
                      tunnel: w844 -> [w849]
                      tunnel: [w849] -> w843
                      tunnel: w843 -> [w851]
                      tunnel: [w855] -> w842
                      tunnel: [w854] -> w841
                      tunnel: [w851] -> w840
                      tunnel: w842 -> [w861]
                      tunnel: w841 -> [w860]
                      tunnel: w840 -> [w856]
                      frame #0 {
                        n242 = property on="Set Gauge to Zero" class="Bool"("Blinking"=TRUE) -> ()  [unwired: 2 in, 2 out]
                      }
                      frame #1 {
                        w852 = 0 items=["sensor 1", "sensor 2", "test"] ("Sensor Nr.:")
                        n243 = call "DUAL GAUGE-Get Pressure,Status.vi"("Sensor Nr.:"=w852, "Referenz in"=w851) -> ("Pressure"=w855:dbl)  [unwired: 6 in, 3 out]
                        n244 = call "DUAL GAUGE-Offset display.vi"("W/R"=FALSE, "Referenz in"=w851) -> ("Sensor 1 Get"=w854:dbl)  [unwired: 6 in, 3 out]
                      }
                      frame #2 {
                        n245 = Add(x=w861, y=w860) -> (x+y=w857:dbl)
                        n246 = call "DUAL GAUGE-Offset display.vi"("W/R"=TRUE, "Sensor 1 Set"=w857, "Referenz in"=w856) -> ("Sensor 1 Get"=→"Current Offset (mbar)":dbl)  [unwired: 5 in, 3 out]
                      }
                      frame #3 {
                        n247 = property on="Set Gauge to Zero" class="Bool"("Blinking"=TRUE) -> ()  [unwired: 2 in, 2 out]
                      }
                    }
                    n248 = Unbundle(w848) -> ("VISA resource name out"=w847:refnum<visa-resource-name>, "error out"=w846:errorcluster)  [unwired: 2 out]
                  }
                  event "Write to File": Value Change {
                    n249 = event-data() -> ("NewVal"=w867:bool)  [unwired: 1 in]
                    n250 = Unbundle(w870) -> ("VISA resource name out"=w869:refnum<visa-resource-name>, "error out"=w868:errorcluster)  [unwired: 2 out]
                    n251 = local read "File Path"() -> (w863:path)
                    n252 = case shown="True" w867 {
                      tunnel: w863 -> [_ w875]
                      tunnel: "User" -> [_ w874]
                      tunnel: "Sample" -> [_ w873]
                      tunnel: [path "" ("File Path") w872] -> w864
                      frame False {
                      }
                      frame True {
                        n253 = call "Header.vi"("Sample"=w873, "User"=w874, "File Path"=w875) -> ("File Path"=w872:path)
                      }
                    }
                    n254 = local write "File Path"(w864) -> ()
                  }
                }
              }
              n255 = Bundle(cluster=w369, "VISA resource name out"=w368, "error out"=w367) -> (w366:T7)  [unwired: 2 in]
            }
            frame #2 {
            }
            frame #3 {
              (unwired) "Daniel Schuster (geb. 20.03.1988)"
              n256 = node-c288(w928) -> (w937:T3)  [unwired: 2 in]
              n257 = node-c288(w943) -> (w946:T3)  [unwired: 2 in]
              n258 = node-c288(w933) -> (w935:T3)  [unwired: 2 in]
              n259 = node-c288(w942) -> (w950:T3)  [unwired: 2 in]
              n260 = timed-sequence {
                timing: w937 -> [_]
                timing-out: [_] -> w936
                tunnel: w912 -> [w993]
                tunnel: w911 -> [w989]
                tunnel: [w992] -> w904
                tunnel: w903 -> [w991]
                tunnel: w902 -> [w990]
                tunnel: [w988] -> w901
                tunnel: [w987] -> w900
                tunnel: [w986] -> w899
                n261 = timed-flat-sequence {
                  tunnel: w993 -> [w1002]
                  tunnel: [w1001] -> w992
                  tunnel: w991 -> [w1000]
                  tunnel: w990 -> [w999]
                  tunnel: w989 -> [w998]
                  tunnel: [w996] -> w988
                  tunnel: [w995] -> w987
                  tunnel: [w994] -> w986
                  n262 = node-c288() -> ()  [unwired: 1 in, 1 out]
                  n263 = case shown="True" "ON (TPG 2)" {
                    tunnel: w998 -> [w1007 w1013]
                    tunnel: w999 -> [w1006 w1012]
                    tunnel: [w1005 w1011] -> w995
                    tunnel: [w1004 w1010] -> w994
                    frame False {
                      w1008 = 0.0 ("Pressure")
                      n264 = property on="ON (TPG 2)" class="Bool (strict)"("Blinking"=FALSE) -> ()  [unwired: 2 in, 2 out]
                      n265 = Bundle("Pressure"=w1008, "Pressure"=w1008) -> (w1005:cluster{"Pressure":dbl, "Pressure":dbl})  [unwired: 1 in]
                      n266 = Bundle("TPG 2 COM"=w1007, "error out"=w1006) -> (w1004:T8)  [unwired: 1 in]
                    }
                    frame True {
                      n267 = stacked-sequence {
                        tunnel: w1013 -> [_ w1026]
                        tunnel: [_ w1022] -> w1011
                        tunnel: [_ w1018] -> w1010
                        tunnel: w1012 -> [_ w1015]
                        frame #0 {
                          n268 = property on="ON (TPG 2)" class="Bool (strict)"("Blinking"=TRUE) -> ()  [unwired: 2 in, 2 out]
                        }
                        frame #1 {
                          n269 = call "PresureGetSubVI.vi"("COM in"=w1026, "Fehler (Eingang)"=w1015) -> ("Status Gauge#1"=→"Status Gauge 2#1":i32, "Status Gauge#2"=→"Status Gauge 2#2":i32, "COM out"=w1019:refnum<visa-resource-name>, "Pressure Gauge#1"=w1020:dbl, "Pressure Gauge#2"=w1023:dbl, "Cluster (Ausgang)"=w1016:errorcluster)  [unwired: 12 in]
                          "Pressure Gauge 2#1" <- w1020
                          "Pressure Gauge 2#2" <- w1023
                          n270 = Bundle("COM out"=w1019, "Cluster (Ausgang)"=w1016) -> (w1018:T9)  [unwired: 1 in]
                          n271 = Unbundle(w1016) -> ("status"=w1017:bool, "code"=w1021:i32)  [unwired: 1 out]
                          n272 = Bundle("status"=w1017, "code"=w1021) -> ()  [unwired: 1 in, 1 out]
                          n273 = Bundle("Pressure Gauge#1"=w1020, "Pressure Gauge#2"=w1023) -> (w1022:T10)  [unwired: 1 in]
                        }
                      }
                    }
                  }
                  n274 = case shown="True" "ON (TPG 1)" {
                    tunnel: w1002 -> [w1030 w1036]
                    tunnel: [w1029 w1035] -> w1001
                    tunnel: w1000 -> [w1028 w1034]
                    tunnel: [w1027 w1033] -> w996
                    frame False {
                      w1031 = 0.0 ("Pressure")
                      n275 = property on="ON (TPG 1)" class="Bool (strict)"("Blinking"=FALSE) -> ()  [unwired: 2 in, 2 out]
                      n276 = Bundle("Pressure"=w1031, "Pressure"=w1031) -> (w1027:cluster{"Pressure":dbl, "Pressure":dbl})  [unwired: 1 in]
                      n277 = Bundle("TPG 1 COM"=w1030, "error out"=w1028) -> (w1029:T11)  [unwired: 1 in]
                    }
                    frame True {
                      n278 = stacked-sequence {
                        tunnel: w1036 -> [_ w1049]
                        tunnel: [_ w1042] -> w1035
                        tunnel: w1034 -> [_ w1039]
                        tunnel: [_ w1038] -> w1033
                        frame #0 {
                          n279 = property on="ON (TPG 1)" class="Bool (strict)"("Blinking"=TRUE) -> ()  [unwired: 2 in, 2 out]
                        }
                        frame #1 {
                          n280 = call "PresureGetSubVI.vi"("COM in"=w1049, "Fehler (Eingang)"=w1039) -> ("Status Gauge#1"=→"Status Gauge 1#1":i32, "Status Gauge#2"=→"Status Gauge 1#2":i32, "COM out"=w1043:refnum<visa-resource-name>, "Pressure Gauge#1"=w1044:dbl, "Pressure Gauge#2"=w1046:dbl, "Cluster (Ausgang)"=w1040:errorcluster)  [unwired: 12 in]
                          "Pressure Gauge 1#1" <- w1044
                          "Pressure Gauge 1#2" <- w1046
                          n281 = Bundle("COM out"=w1043, "Cluster (Ausgang)"=w1040) -> (w1042:T9)  [unwired: 1 in]
                          n282 = Unbundle(w1040) -> ("status"=w1041:bool, "code"=w1045:i32)  [unwired: 1 out]
                          n283 = Bundle("status"=w1041, "code"=w1045) -> ()  [unwired: 1 in, 1 out]
                          n284 = Bundle("Pressure Gauge#1"=w1044, "Pressure Gauge#2"=w1046) -> (w1038:T10)  [unwired: 1 in]
                        }
                      }
                    }
                  }
                  n285 = node-c288() -> ()  [unwired: 1 in, 1 out]
                }
              }
              n286 = timed-sequence {
                timing: w946 -> [_]
                timing-out: [_] -> w945
                tunnel: w944 -> [w1059]
                tunnel: [w1058] -> w939
                tunnel: [w1057] -> w938
                tunnel: [w1056] -> w925
                n287 = timed-flat-sequence {
                  tunnel: w1059 -> [w1063]
                  tunnel: [w1062] -> w1058
                  tunnel: [w1061] -> w1057
                  tunnel: [w1060] -> w1056
                  n288 = node-c288() -> ()  [unwired: 1 in, 1 out]
                  n289 = case shown="True" "ON" {
                    tunnel: w1063 -> [w1067 w1072]
                    tunnel: [w1066 w1071] -> w1062
                    tunnel: [w1065 w1070] -> w1061
                    tunnel: [_ w1069] -> w1060
                    frame False {
                      n290 = Unbundle(w1067) -> ("VISA resource name out"=w1066:refnum<visa-resource-name>, "error out"=w1065:errorcluster)  [unwired: 2 out]
                      n291 = property on="ON" class="Bool (strict)"("Blinking"=FALSE) -> ()  [unwired: 2 in, 2 out]
                    }
                    frame True {
                      n292 = stacked-sequence {
                        tunnel: w1072 -> [_ w1077]
                        tunnel: [_ w1076] -> w1071
                        tunnel: [_ w1075] -> w1070
                        tunnel: [_ w1074] -> w1069
                        frame #0 {
                          n293 = property on="ON" class="Bool (strict)"("Blinking"=TRUE) -> ()  [unwired: 2 in, 2 out]
                        }
                        frame #1 {
                          n294 = Unbundle(w1077) -> ("VISA resource name out"=w1081:refnum<visa-resource-name>, "error out"=w1079:errorcluster, "Delay (ms)"=w1080:u32, "Write/\nRead"=w1078:bool)
                          n295 = call "I3252_Comm_Interface.vi"("VISA resource name in"=w1081, "error in"=w1079, "Delay (ms)"=w1080, "Write"=w1078, "String to Write"="*V01", "Read"=w1078) -> ("VISA resource name out"=w1076:refnum<visa-resource-name>, "error out"=w1075:errorcluster, "Read String"=w1074:string)  [unwired: 2 in]
                        }
                      }
                    }
                  }
                  n296 = node-c288() -> ()  [unwired: 1 in, 1 out]
                }
              }
              n297 = timed-sequence {
                timing: w935 -> [_]
                timing-out: [_] -> w934
                tunnel: w932 -> [w955]
                tunnel: w931 -> [w954]
                tunnel: [w953] -> w929
                tunnel: [w952] -> w930
                tunnel: [w951] -> w926
                n298 = timed-flat-sequence {
                  tunnel: w955 -> [w960]
                  tunnel: w954 -> [w959]
                  tunnel: [w958] -> w953
                  tunnel: [w957] -> w952
                  tunnel: [w956] -> w951
                  n299 = node-c288() -> ()  [unwired: 1 in, 1 out]
                  n300 = case shown="False" "ON" {
                    tunnel: w960 -> [w964 w970]
                    tunnel: w959 -> [w965 w969]
                    tunnel: [w964 w968] -> w958
                    tunnel: [w965 w967] -> w957
                    tunnel: [0.0 ("Reading") w966] -> w956
                    frame False {
                      n301 = property on="ON" class="Bool (strict)"("Blinking"=FALSE) -> ()  [unwired: 2 in, 2 out]
                    }
                    frame True {
                      n302 = stacked-sequence {
                        tunnel: w970 -> [_ w977]
                        tunnel: w969 -> [_ w976]
                        tunnel: [_ w975] -> w968
                        tunnel: [_ w974] -> w967
                        tunnel: [_ w972] -> w966
                        frame #0 {
                          n303 = property on="ON" class="Bool (strict)"("Blinking"=TRUE) -> ()  [unwired: 2 in, 2 out]
                        }
                        frame #1 {
                          n304 = call "VC840_Read.vi"("error in (no error)"=w976, "VISA resource name"=w977) -> ("error out"=w974:errorcluster, "Unit"=→"Unit 2":string, "Reading"=w972:dbl, "VISA resource name out"=w975:refnum<visa-resource-name>, "Status"=→"Status 2":T2, "Mode"=→"Mode 2":enum16{"?", "Diode", "Beep", "DC", "AC"})  [unwired: 4 out]
                          "Reading 2" <- w972
                        }
                      }
                    }
                  }
                  n305 = node-c288() -> ()  [unwired: 1 in, 1 out]
                }
              }
              n306 = timed-sequence {
                timing: w950 -> [_]
                timing-out: [_] -> w949
                tunnel: w948 -> [w1093]
                tunnel: w947 -> [w1092]
                tunnel: [w1091] -> w941
                tunnel: [w1090] -> w940
                tunnel: [w1089] -> w927
                n307 = timed-flat-sequence {
                  tunnel: w1093 -> [w1098]
                  tunnel: w1092 -> [w1097]
                  tunnel: [w1096] -> w1091
                  tunnel: [w1095] -> w1090
                  tunnel: [w1094] -> w1089
                  n308 = node-c288() -> ()  [unwired: 1 in, 1 out]
                  n309 = case shown="True" "ON" {
                    tunnel: w1098 -> [w1102 w1108]
                    tunnel: w1097 -> [w1103 w1107]
                    tunnel: [w1102 w1106] -> w1096
                    tunnel: [w1103 w1105] -> w1095
                    tunnel: [0.0 ("Reading") w1104] -> w1094
                    frame False {
                      n310 = property on="ON" class="Bool (strict)"("Blinking"=FALSE) -> ()  [unwired: 2 in, 2 out]
                    }
                    frame True {
                      n311 = stacked-sequence {
                        tunnel: w1108 -> [_ w1115]
                        tunnel: w1107 -> [_ w1114]
                        tunnel: [_ w1113] -> w1106
                        tunnel: [_ w1112] -> w1105
                        tunnel: [_ w1110] -> w1104
                        frame #0 {
                          n312 = property on="ON" class="Bool (strict)"("Blinking"=TRUE) -> ()  [unwired: 2 in, 2 out]
                        }
                        frame #1 {
                          n313 = call "VC840_Read.vi"("error in (no error)"=w1114, "VISA resource name"=w1115) -> ("error out"=w1112:errorcluster, "Unit"=→"Unit 1":string, "Reading"=w1110:dbl, "VISA resource name out"=w1113:refnum<visa-resource-name>, "Status"=→"Status 1":T2, "Mode"=→"Mode 1":enum16{"?", "Diode", "Beep", "DC", "AC"})  [unwired: 4 out]
                          "Reading 1" <- w1110
                        }
                      }
                    }
                  }
                  n314 = node-c288() -> ()  [unwired: 1 in, 1 out]
                }
              }
              n315 = Tick Count (ms)() -> (millisecond timer value=w913:u32)
              n316 = Subtract(x=w913, y=w918) -> (x-y=w917:u32)
              n317 = Divide(x=w917, y=u32 1000) -> (x/y=w915:dbl)
              n318 = node-c288(w949) -> ()  [unwired: 1 out]
              n319 = node-c288(w934) -> ()  [unwired: 1 out]
              n320 = node-c288(w945) -> ()  [unwired: 1 out]
              n321 = To Double Precision Float(number=w915) -> (double precision float=w919:dbl)
              "current time (s)" <- w919
              n322 = node-c288(w936) -> ()  [unwired: 1 out]
              n323 = Unbundle(w900) -> ("Pressure Gauge#1"=w897:dbl, "Pressure Gauge#2"=w898:dbl)
              "Pressure Gauge 2#2" <- w898
              "Pressure Gauge 2#1" <- w897
              n324 = Unbundle(w901) -> ("Pressure Gauge#1"=w910:dbl, "Pressure Gauge#2"=w905:dbl)
              "Pressure Gauge 1#1" <- w910
              "Pressure Gauge 1#2" <- w905
            }
            frame #4 {
              n325 = Build Array (concatenate)(w1135, w1139) -> (w1134:dbl[])
              n326 = Build Array (concatenate)(w1138, w1140) -> (w1133:dbl[])
              n327 = Build Array (concatenate)(w1136, w1127) -> (w1131:dbl[])
              n328 = Build Array (concatenate)(w1137, w1128) -> (w1132:dbl[])
              n329 = Greater?(x=w1159, y="Pressure Limit (mbar)") -> (0:w1162:bool)
              n330 = case shown="False" w1162 {
                frame False {
                  n331 = property on="Standby" class="Bool (strict)"("DisabledEnum"=T6."Enabled" ("Disabled")) -> ()  [unwired: 2 in, 2 out]
                }
                frame True {
                  n332 = property on="Standby" class="Bool (strict)"("Val(Sgnl)"=TRUE ("Standby"), "DisabledEnum"=T6."Disabled" ("Disabled")) -> ()  [unwired: 2 in, 2 out]
                }
              }
              n333 = call "Resistivity_Calculation.vi"("Reading 1 (V)"=w1152, "Constant"="4PP constant", "Thickness (nm)"="Thickness (nm)", "Reading 2 (A)"=w1160) -> ("Resivtivity (Ohm*cm)"=w1144:dbl, "Current"=w1145:dbl, "Voltage"=w1146:dbl)
              "Resistivity (Ohm*cm)" <- w1144
              "Voltage (V)" <- w1146
              "Current (A)" <- w1145
              n334 = call "I3252_Edit_Temperature.vi"("Temp. String"=w1161) -> ("Temp. (°C)"=w1155:dbl)
              "(°C)" <- w1155
              n335 = Build Array (concatenate)(w1157, w1158) -> (w1154:dbl[])
              n336 = Build Array (concatenate)(w1156, w1155) -> (w1142:dbl[])
              n337 = Build Array (concatenate)(w1153, w1146) -> (w1151:dbl[])
              n338 = Build Array (concatenate)(w1150, w1145) -> (w1148:dbl[])
              n339 = Build Array (concatenate)(w1149, w1144) -> (w1147:dbl[])
              n340 = Build Array(w1146, w1145, w1144) -> (w1143:dbl[])
            }
            frame #5 {
              n341 = Bundle(w1190, w1189) -> (→"Main Chamber (PG-1)":cluster{dbl[], dbl[]})  [unwired: 1 in]
              n342 = Bundle(w1190, w1188) -> (→"Loadlock (PG-3)":cluster{dbl[], dbl[]})  [unwired: 1 in]
              n343 = Bundle(w1190, w1187) -> (→"Pirani (VVP1 Scroll)":cluster{dbl[], dbl[]})  [unwired: 1 in]
              n344 = Bundle(w1190, w1186) -> (→"Pressure OpenPort":cluster{dbl[], dbl[]})  [unwired: 1 in]
              n345 = Bundle(w1190, w1196) -> (→"Sample holder (Type-K Thermocouple)":cluster{dbl[], dbl[]})  [unwired: 1 in]
              n346 = Bundle(w1190, w1198) -> (→"Voltage":cluster{dbl[], dbl[]})  [unwired: 1 in]
              n347 = Bundle(w1190, w1199) -> (→"Current":cluster{dbl[], dbl[]})  [unwired: 1 in]
              n348 = Bundle(w1190, w1200) -> (→"Resistivity":cluster{dbl[], dbl[]})  [unwired: 1 in]
              n349 = Build Array (concatenate)(w1195, w1205, w1204, w1194, w1181, w1178, w1176) -> (w1212:dbl[])
              "appended array" <- w1212
            }
            frame #6 {
              n350 = Unbundle(w1218) -> ("COM out"=w1217:refnum<visa-resource-name>, "Cluster (Ausgang)"=w1216:errorcluster)
              n351 = Unbundle(w1215) -> ("COM out"=w1214:refnum<visa-resource-name>, "Cluster (Ausgang)"=w1213:errorcluster)
              n352 = case shown="True" "Write to File" {
                tunnel: [_ w1246] -> w1232
                tunnel: "File Path" -> [_ w1244]
                tunnel: w1225 -> [_ w1242]
                frame False {
                  n353 = property on="Write to File" class="Bool (strict)"("Blinking"=FALSE) -> ()  [unwired: 2 in, 2 out]
                }
                frame True {
                  n354 = flat-sequence {
                    tunnel: [w1248] -> w1245
                    tunnel: w1244 -> [w1248]
                    tunnel: [w1247] -> w1243
                    tunnel: w1242 -> [w1247]
                    tunnel: [w1253] -> w1246
                    tunnel: w1245 -> [w1252]
                    tunnel: w1243 -> [w1251]
                    frame #0 {
                      n355 = property on="Write to File" class="Bool (strict)"("Blinking"=TRUE) -> ()  [unwired: 2 in, 2 out]
                    }
                    frame #1 {
                      n356 = call-poly <vilib>:"Write To Spreadsheet File.vi"("format (%.3f)"="%g", "append to file? (new file:F)"=TRUE ("transpose? (no:F)"), "1D data"=w1251, "file path (dialog if empty)"=w1252) -> ("new file path (Not A Path if cancelled)"=w1253:path)  [unwired: 4 in]
                    }
                  }
                }
              }
              n357 = Merge Errors(w1237, w1236, w1234, w1216, w1213) -> (w1235:errorcluster)
              n358 = call <vilib>:"Simple Error Handler.vi"("error in (no error)"=w1235) -> ("error?"=w1219:bool)  [unwired: 4 in, 4 out]
              n359 = local write "File Path"(w1232) -> ()
            }
            frame #7 {
              w1270 = u32 1000 ("y")
              n360 = Tick Count (ms)() -> (millisecond timer value=w1272:u32)
              n361 = Subtract(x=w1272, y=w1271) -> (x-y=w1273:u32)
              n362 = VISA Flush I/O Buffer(VISA resource name=w1265, error in (no error)=w1264) -> (VISA resource name out=w1262:refnum<visa-resource-name>, error out=w1263:errorcluster)  [unwired: 1 in]
              n363 = VISA Flush I/O Buffer(VISA resource name=w1258, error in (no error)=w1257) -> (VISA resource name out=w1261:refnum<visa-resource-name>, error out=w1260:errorcluster)  [unwired: 1 in]
              n364 = Divide(x=w1273, y=w1270) -> (x/y=w1256:ext)
              "loop time (s)" <- w1256
              n365 = Subtract(x="Intervall (s)", y=w1256) -> (x-y=w1255:ext)
              n366 = Multiply(x=w1255, y=w1270) -> (x*y=w1275:ext)
              n367 = Wait (ms)(milliseconds to wait=w1275) -> ()  [unwired: 1 out]
              n368 = Bundle("COM out"=w1262, "error out"=w1263, "COM out"=w1261, "error out"=w1260) -> (w1259:T12)  [unwired: 1 in]
            }
            frame #8 {
              n369 = Tick Count (ms)() -> (millisecond timer value=w1295:u32)
              n370 = Subtract(x=w1295, y=w1293) -> (x-y=w1294:u32)
              n371 = Divide(x=w1294, y=w1292) -> (x/y=→"data logger intervall (s)":dbl)
            }
          }
          n372 = Exclusive Or(1:"stop", 2:w133) -> (0:w134:bool)
        }
      }
      frame #4 {
        n373 = call "VC840_Close.vi"("error in (no error)"=w1314, "VISA resource name"=w1315) -> ("error out"=w1323:errorcluster)  [unwired: 9 in]
        n374 = call "VC840_Close.vi"("error in (no error)"=w1316, "VISA resource name"=w1317) -> ("error out"=w1321:errorcluster)  [unwired: 9 in]
        n375 = VISA Close(VISA resource name=w1319, error in (no error)=w1318) -> (error out=w1320:errorcluster)
        n376 = Unbundle(w1312) -> ("COM out"=w1311:refnum<visa-resource-name>, "error out"=w1310:errorcluster, "COM out"=w1308:refnum<visa-resource-name>, "error out"=w1309:errorcluster)
        n377 = VISA Close(VISA resource name=w1311, error in (no error)=w1310) -> ()  [unwired: 1 out]
        n378 = VISA Close(VISA resource name=w1308, error in (no error)=w1309) -> ()  [unwired: 1 out]
        n379 = Merge Errors(w1320, w1321, w1323) -> (w1322:errorcluster)
        n380 = call <vilib>:"Simple Error Handler.vi"("error in (no error)"=w1322) -> ("error?"=w1313:bool)  [unwired: 1 in, 7 out]
        n381 = Stop(stop? (T)=w1313) -> ()
      }
    }
  }
